vi "Autonomous Independent.vi"   [LabVIEW 2019]
doc: "This VI is called when autonomous begins, and will automatically be terminated when autonomous ends. You can carry out timed or sensor driven robot movement independently without needing to return to the caller."
uses:
  <vilib>/Rock Robotics/WPI/ThirdParty/Phoenix-LabVIEW/Motor Controller/Sensor/CTRE_Phoenix_MotorControl_SetIntegratedSensorPosition_TalonFX.vi
  <vilib>/Rock Robotics/WPI/Solenoid/WPI_SolenoidValue.ctl
  <vilib>/Rock Robotics/WPI/Solenoid/WPI_SolenoidSetEnum.vi
  <vilib>/Rock Robotics/WPI/ThirdParty/Phoenix-LabVIEW/Motor Controller/Controls/CTRE_Phoenix_MotorControl_ControlMode.ctl
  <vilib>/Rock Robotics/Network Tables/NT Write Number.vi
  <vilib>/Rock Robotics/Network Tables/NT Write Numeric Array.vi
  <vilib>/Rock Robotics/Network Tables/NT Read String.vi
panel:
  # "Be sure to right-click and choose Data Operations>>Make Current Value default if you want to save the array values with the VI"
types:
  T1 = typedef "WPI_JoystickDevRef.ctl" = cluster{"Device":T2}
  T2 = typedef "WPI_JoystickDeviceEnum.ctl" = enum16{"USB 0", "USB 1", "USB 2", "USB 3", "USB 4", "USB 5"}
  T3 = typedef "WPI_MotorControlDeviceRef.ctl" = cluster{"DeviceStatus":errorcluster, "Type":T4, "PWM":cluster{"PWM Channel":T5, "DeadBand":T6}, "CAN":cluster{"Device Number":u8, "SetOutput VI Ref":variant, "GetOutput VI Ref":variant, "Enable VI Ref":variant, "Disable VI Ref":variant, "Data":variant}, "Invert":bool, "DIO PWM":cluster{"PWM \"Enable\" Channel":T5, "DIOChannel":T7, "PWM Rate":dbl}}
  T4 = typedef "WPI_MotorControlType.ctl" = enum16{"PWM", "CAN", "DIO PWM"}
  T5 = typedef "FPGA_DIOPWMChannel.ctl" = enum8{"PWM 0", "PWM 1", "PWM 2", "PWM 3", "PWM 4", "PWM 5", "PWM 6", "PWM 7", "PWM 8", "PWM 9", "PWM MXP 0", "PWM MXP 1", "PWM MXP 2", "PWM MXP 3", "PWM MXP 4", "PWM MXP 5", "PWM MXP 6", "PWM MXP 7", "PWM MXP 8", "PWM MXP 9", "Invalid"}
  T6 = typedef "WPI_PWMDeadband.ctl" = cluster{"Name":string, "maxPositivePwm":i32, "minPositivePwm":i32, "centerPwm":i32, "maxNegativePwm":i32, "minNegativePwm":i32, "angularRange":u16}
  T7 = typedef "FPGA_DIOChannel.ctl" = enum8{"DIO 0", "DIO 1", "DIO 2", "DIO 3", "DIO 4", "DIO 5", "DIO 6", "DIO 7", "DIO 8", "DIO 9", "DIO MXP 0", "DIO MXP 1", "DIO MXP 2", "DIO MXP 3", "DIO MXP 4", "DIO MXP 5", "DIO MXP 6", "DIO MXP 7", "DIO MXP 8", "DIO MXP 9", "DIO MXP 10", "DIO MXP 11", "DIO MXP 12", "DIO MXP 13", "DIO MXP 14", "DIO MXP 15", "SPI Port CS1", "SPI Port CS2", "SPI Port CS3", "SPI Port MISO", "SPI Port MOSI", "Invalid"}
  T8 = typedef "WPI_SolenoidDevRef.ctl" = cluster{"DevStatus":errorcluster, "Pneumatics Control Module":u8, "Forward Solenoid Channel":T9, "Reverse Solenoid Channel":T9}
  T9 = typedef "WPI_SolenoidChannel.ctl" = enum8{"Solenoid 0", "Solenoid 1", "Solenoid 2", "Solenoid 3", "Solenoid 4", "Solenoid 5", "Solenoid 6", "Solenoid 7", "Invalid"}
  T10 = typedef "WPI_SolenoidValue.ctl" = enum16{"Off", "On", "Forward", "Reverse"}
  T11 = typedef "CTRE_Phoenix_MotorControl_ControlMode.ctl" = u16
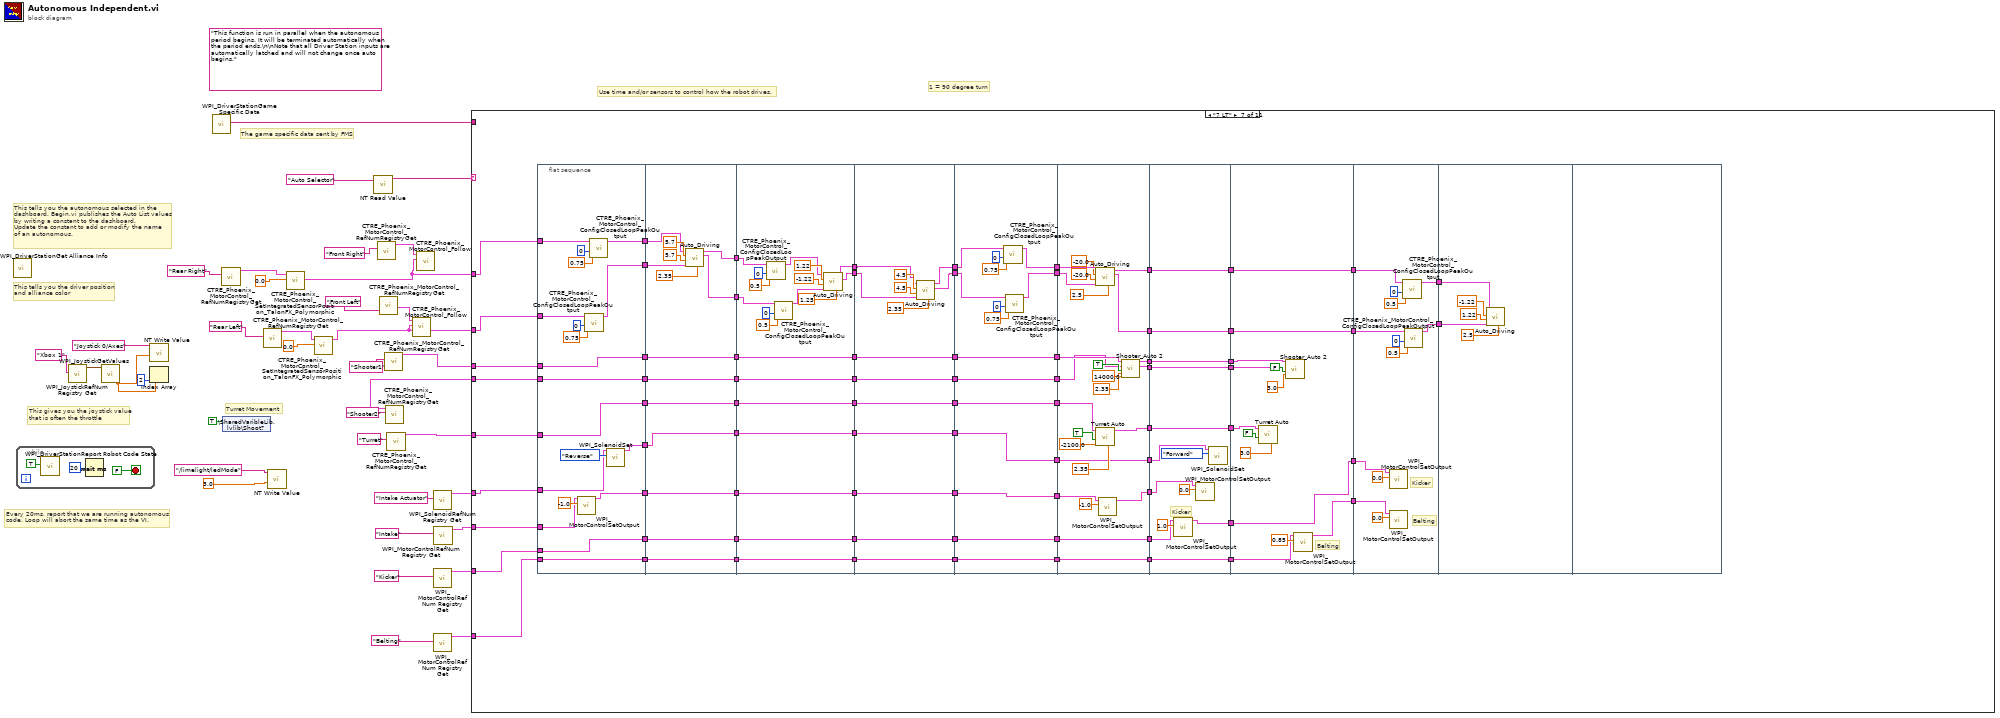
[diagram p0: block diagram]
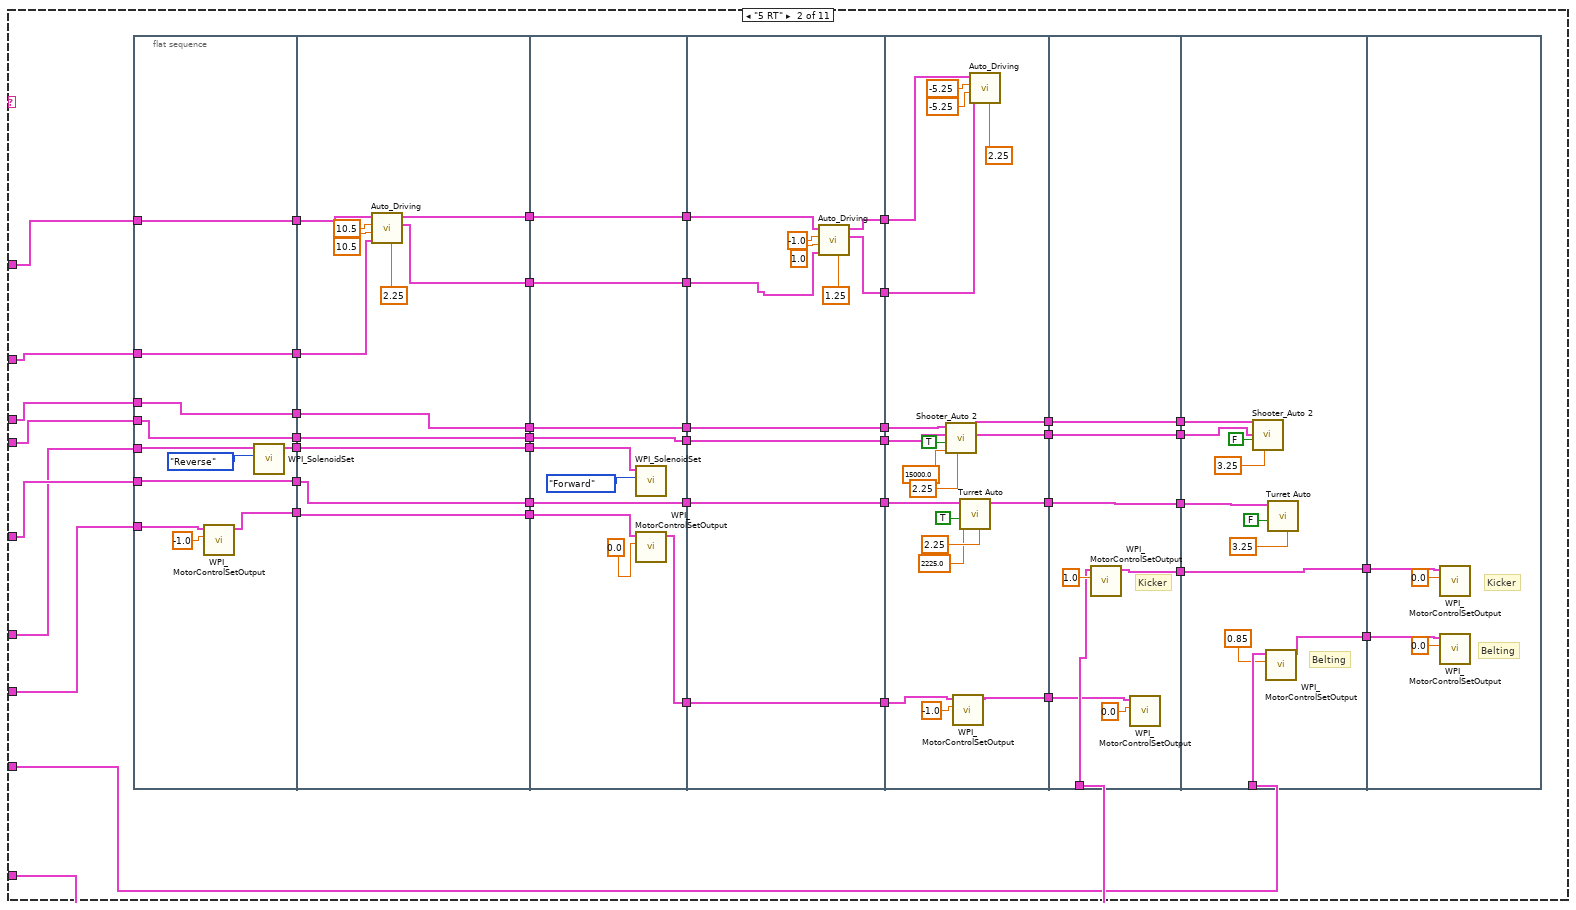
[diagram p3: hidden frame]
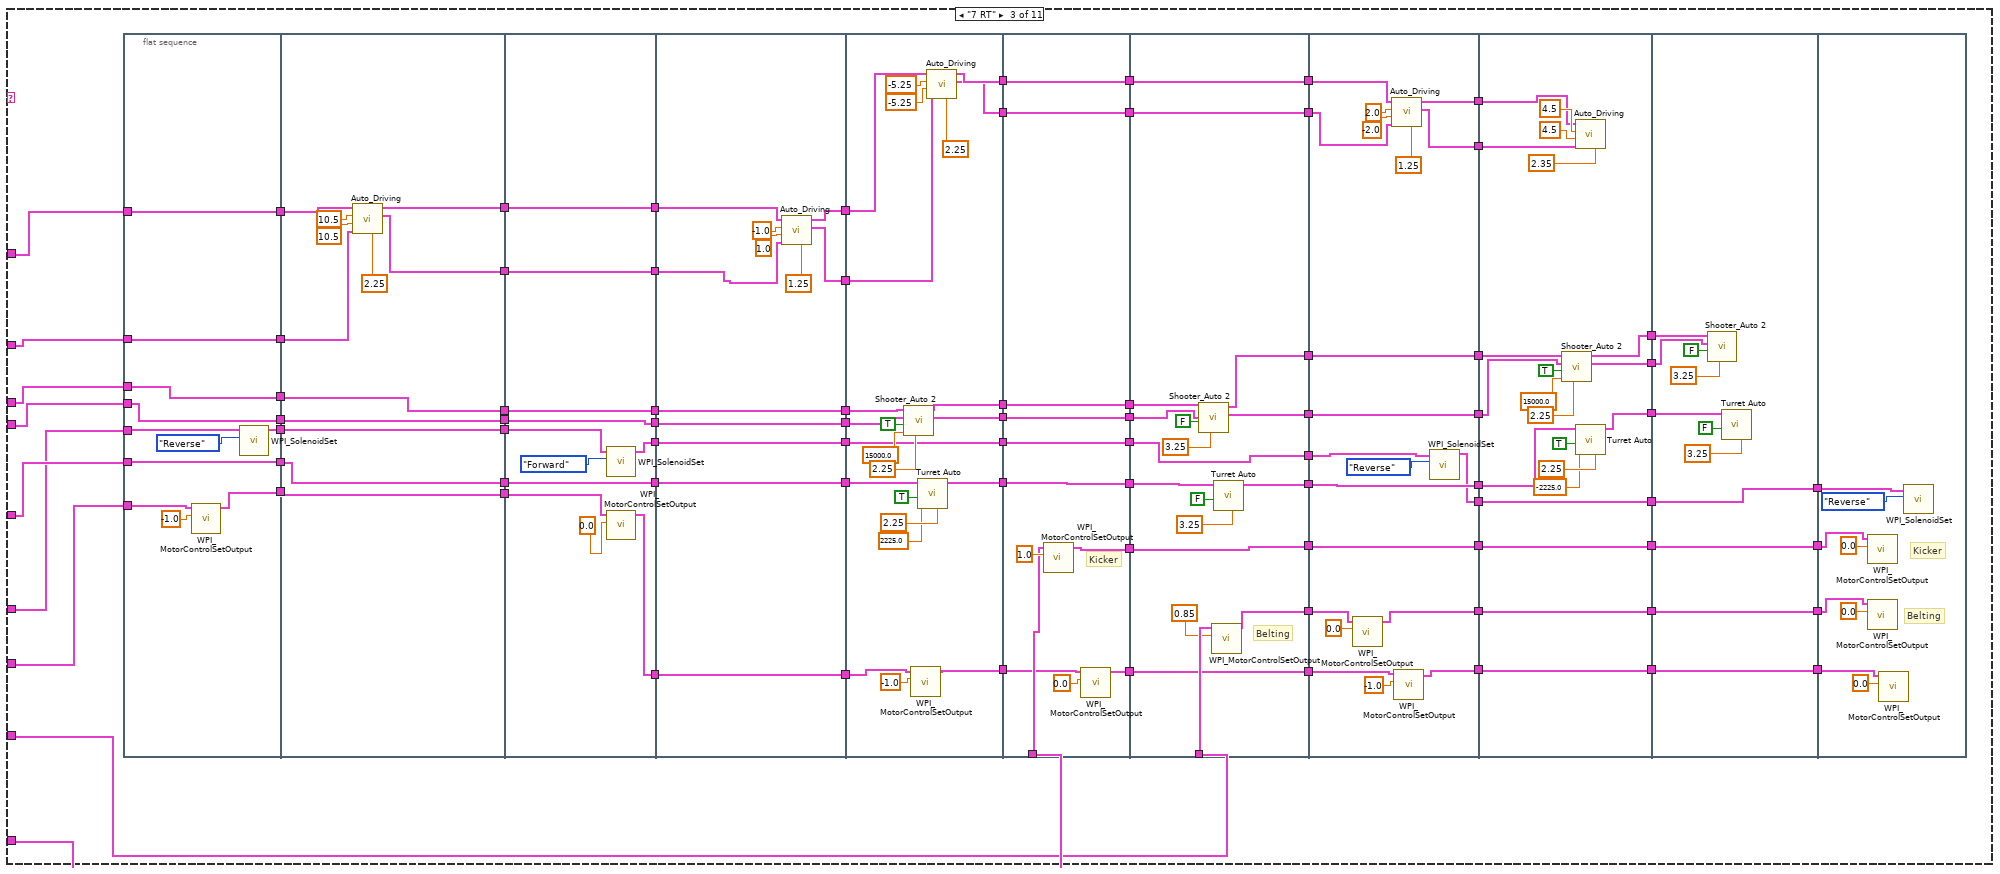
[diagram p4: hidden frame]
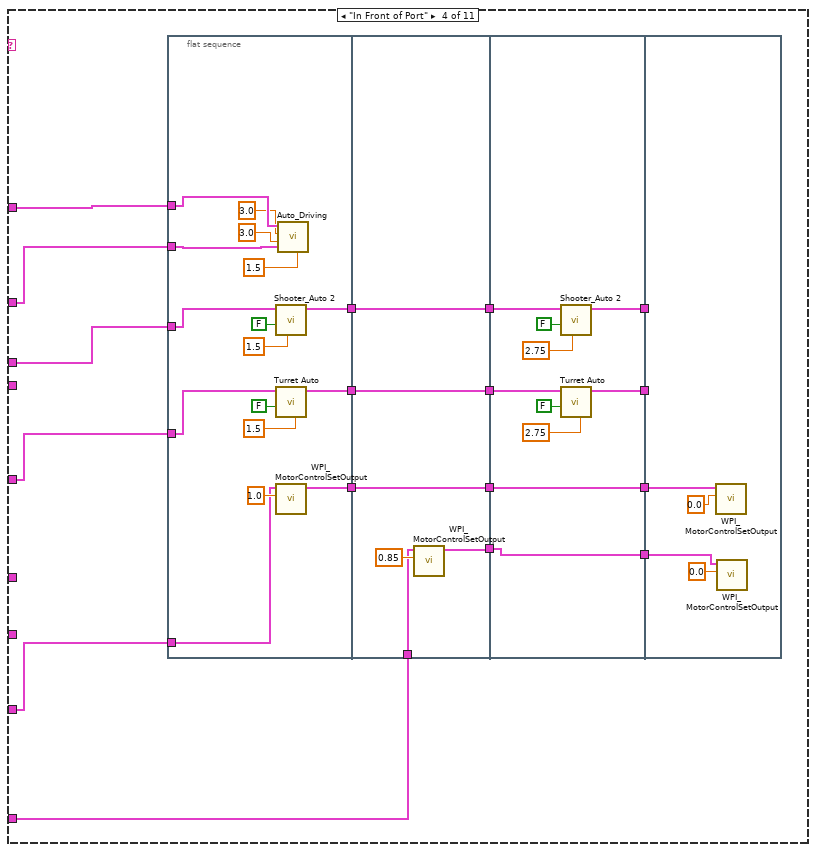
[diagram p5: hidden frame]
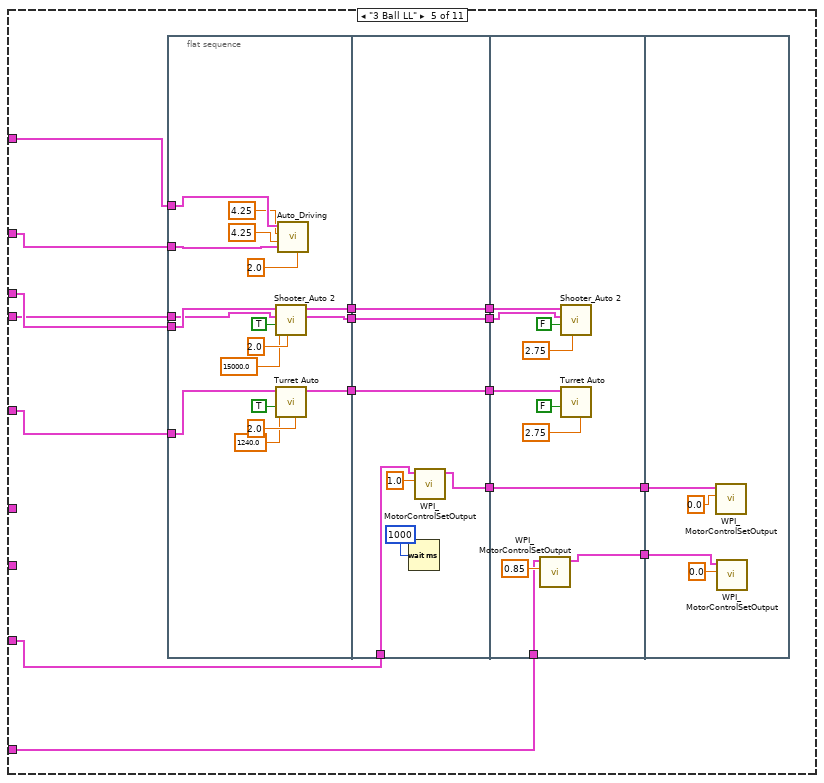
[diagram p6: hidden frame]
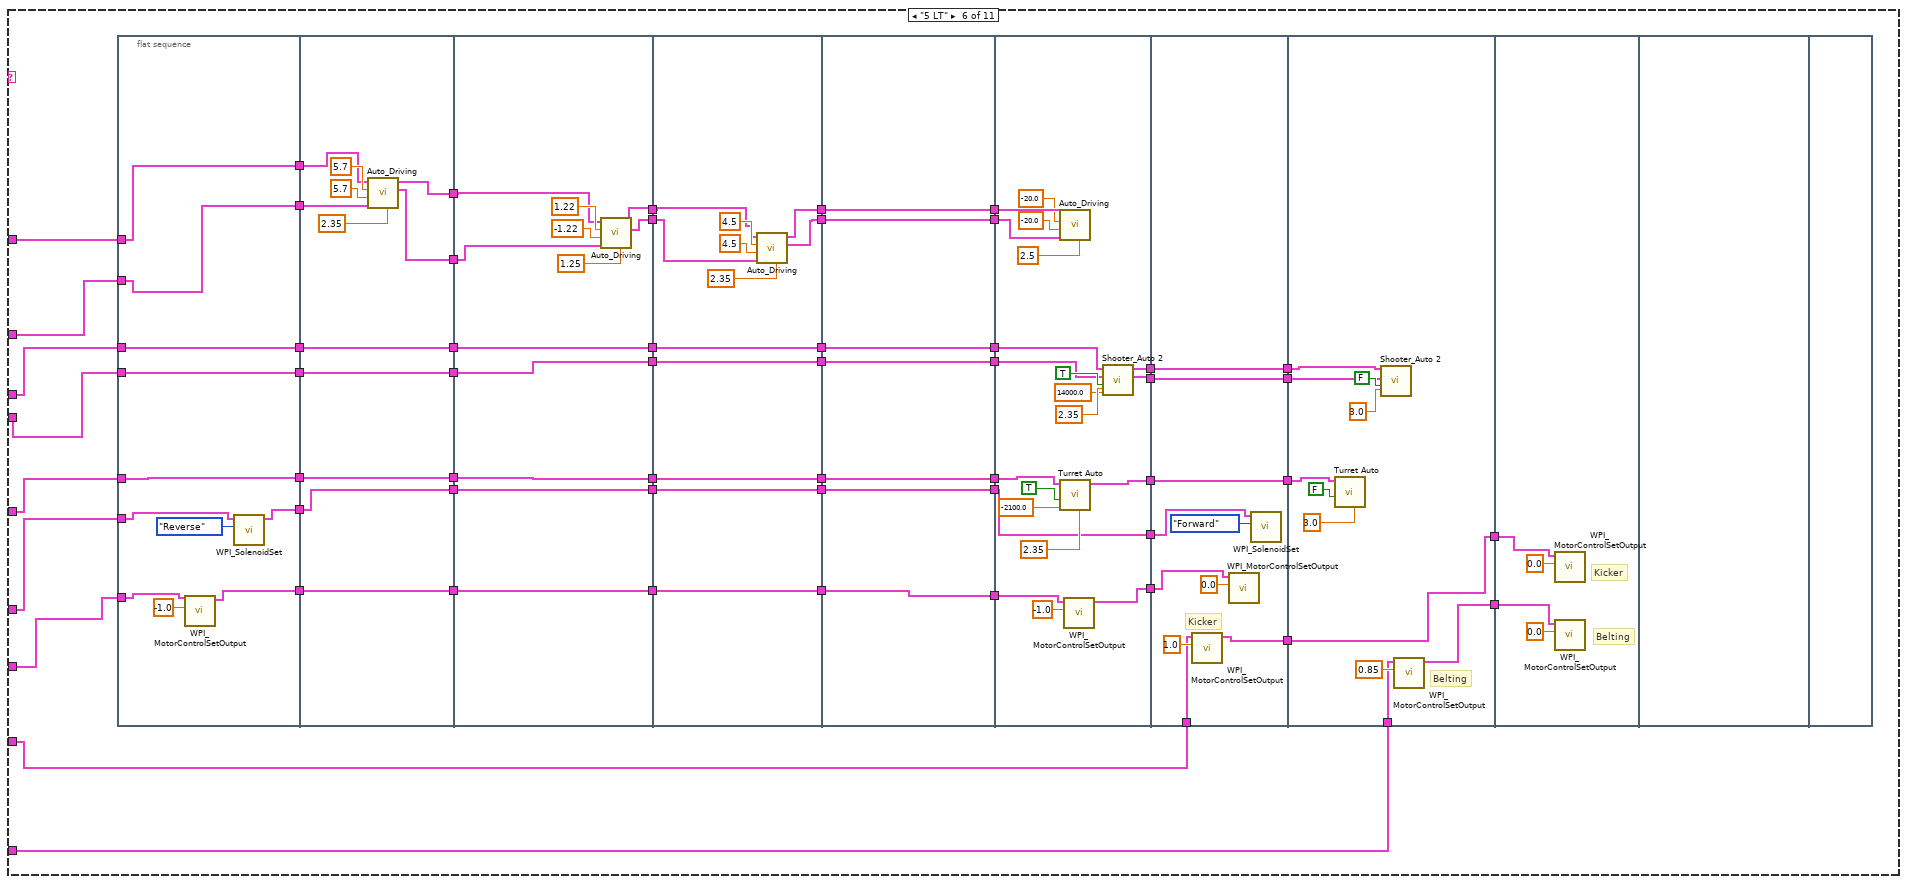
[diagram p7: hidden frame]
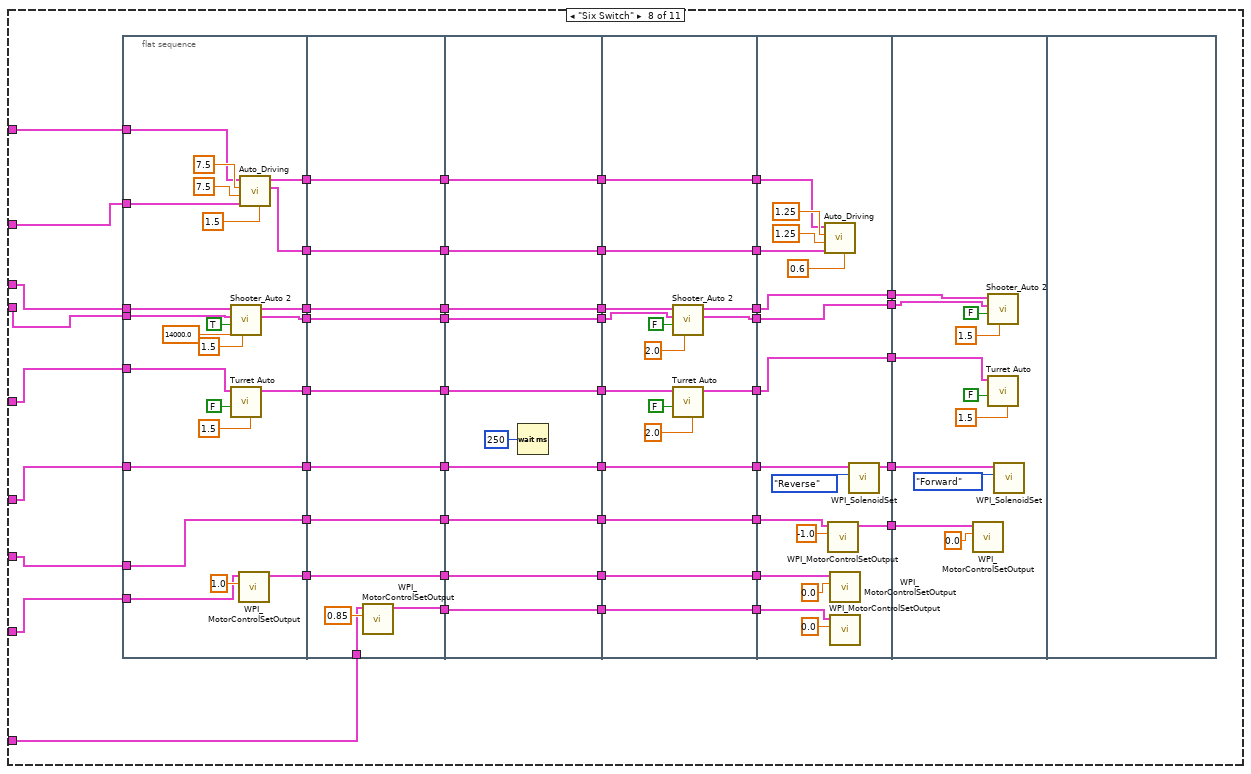
[diagram p8: hidden frame]
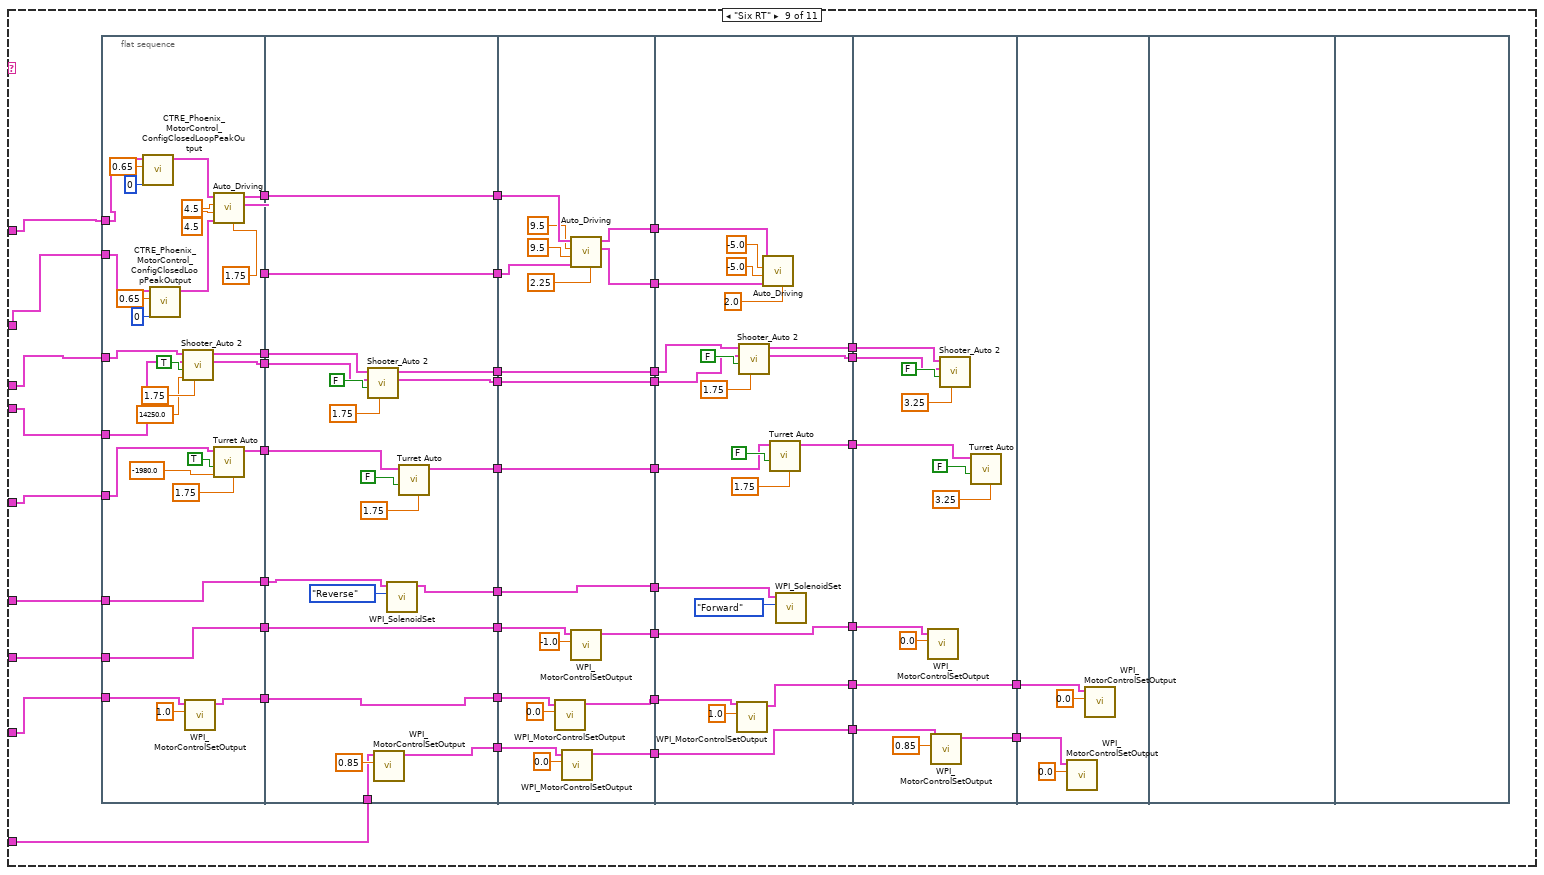
[diagram p9: hidden frame]
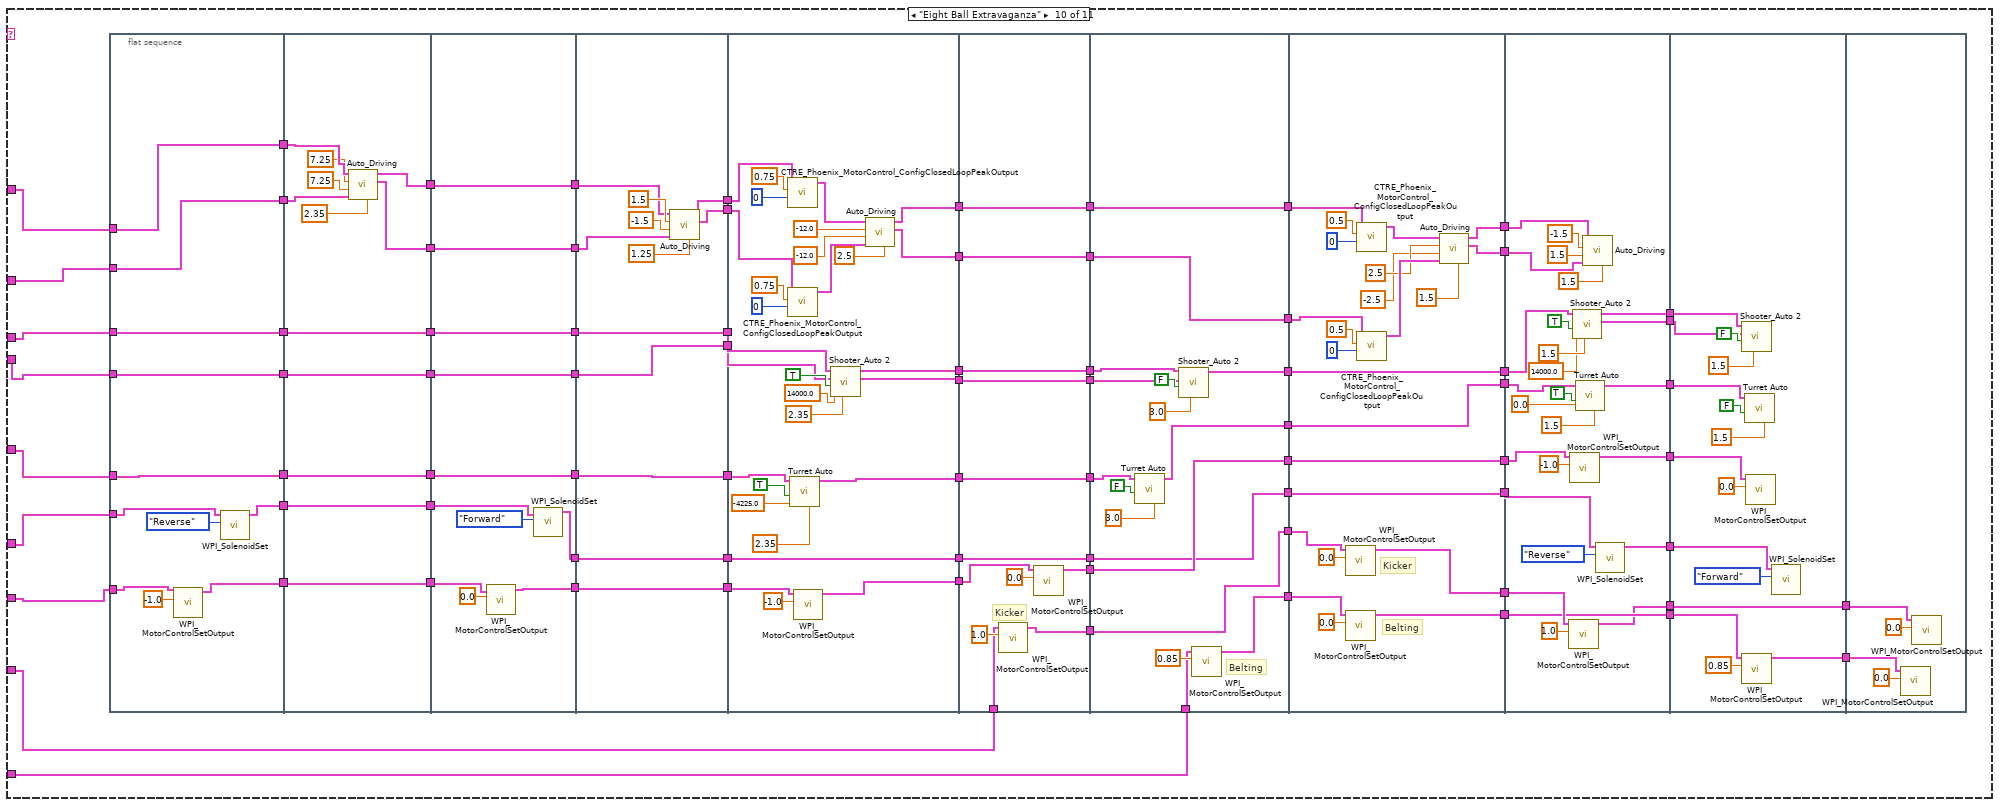
[diagram p10: hidden frame]
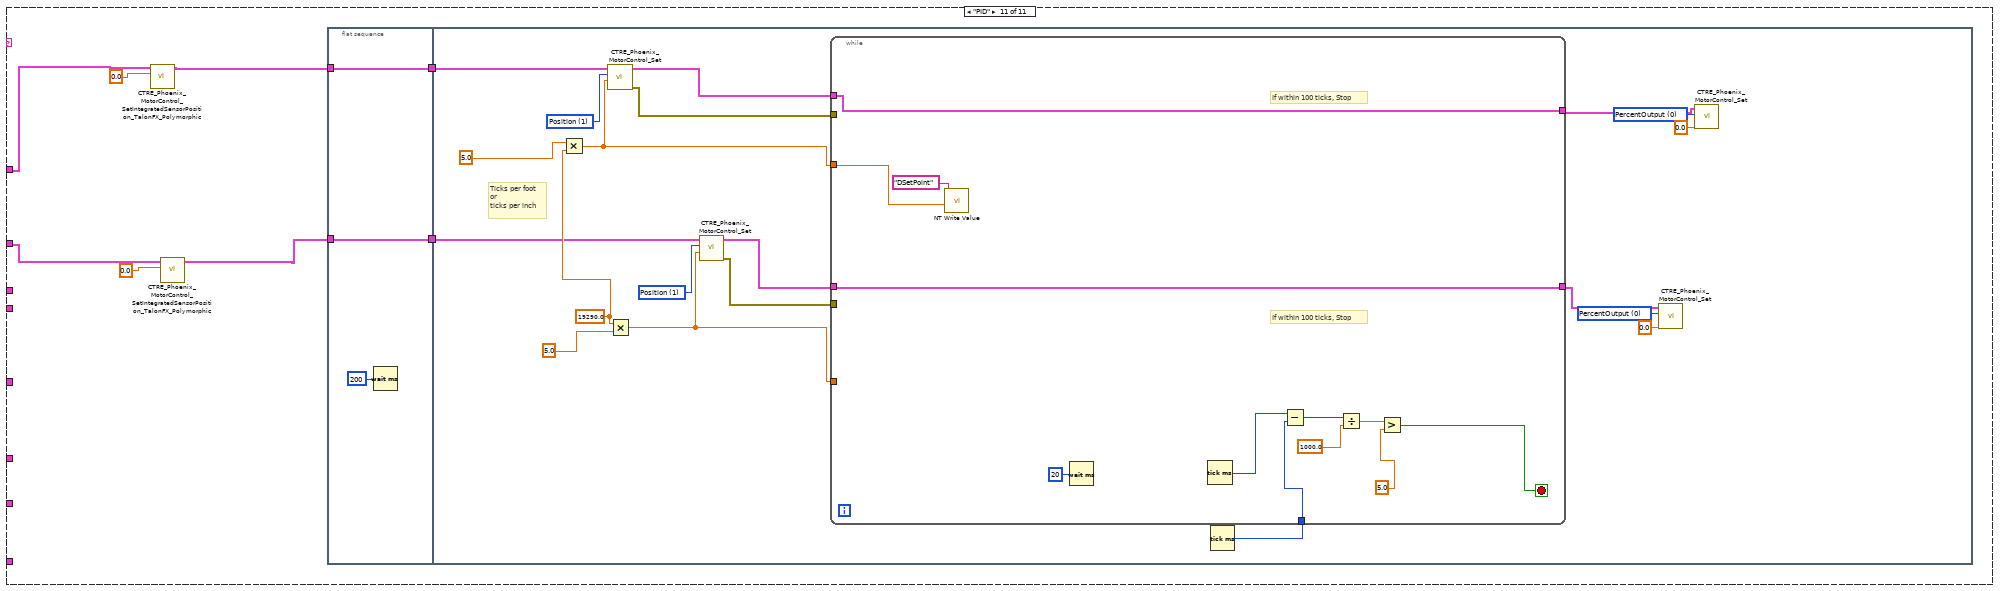
[diagram p11: hidden frame]
diagram:
  (unwired) "This function is run in parallel when the autonomous period begins. It will be terminated automatically when the period ends.\n\nNote that all Driver Station inputs are automatically latched and will not change once auto begins."
  # "1 = 90 degree turn"
  # "Turret Movement"
  # "The game specific data sent by FMS"
  # "This tells you the autonomous selected in the \ndashboard. Begin.vi publishes the Auto List values\nby writing a constant to the dashboard.\nUpdate the constant to add or modify the name\nof an autonomous."
  # "Every 20ms, report that we are running autonomous\ncode. Loop will abort the same time as the VI."
  # "This gives you the joystick value\nthat is often the throttle"
  # "Use time and/or sensors to control how the robot drives."
  # "This tells you the driver position\nand alliance color"
  n1 = call <vilib>:"WPI_DriverStationGet Alliance Info.vi"() -> ()  [unwired: 12 out]
  n2 = while {
    stop <- FALSE stop-if-true
    n3 = call <vilib>:"WPI_DriverStationReport Robot Code State.vi"("Autonomous"=TRUE) -> ()  [unwired: 10 in, 1 out]
    n4 = Wait (ms)(milliseconds to wait=u32 20) -> ()  [unwired: 1 out]
  }
  n5 = call <vilib>:"WPI_JoystickRefNum Registry Get.vi"("refnum name"="Xbox 1") -> ("JoystickDevRef"=w36:T1)  [unwired: 1 in, 9 out]
  n6 = call <vilib>:"WPI_JoystickGetValues.vi"("JoystickDevRef"=w36) -> ("Axes"=w32:dbl[])  [unwired: 6 in, 4 out]
  n7 = call-poly <vilib>:"NT Write Value.vi"("Numeric Array"=w32, "Name"="Joystick 0/Axes") -> ()  [unwired: 9 in, 1 out]
  n8 = Index Array(array=w32, index=2) -> ()  [unwired: 1 out]
  n9 = call <vilib>:"WPI_DriverStationGame Specific Data.vi"() -> ("Game Specific Data"=w30:string)  [unwired: 11 in]
  n10 = call <vilib>:"CTRE_Phoenix_MotorControl_RefNumRegistryGet.vi"("refnum name"="Rear Right") -> ("PhoenixMotorControlDevRef"=w15:T3)  [unwired: 9 in, 1 out]
  n11 = shared-variable ".\\SharedVaribleLib.lvlib\\Shoot?"(TRUE ("Shoot?")) -> ()  [unwired: 1 in, 1 out]
  n12 = call <vilib>:"CTRE_Phoenix_MotorControl_RefNumRegistryGet.vi"("refnum name"="Rear Left") -> ("PhoenixMotorControlDevRef"=w18:T3)  [unwired: 9 in, 1 out]
  n13 = call-poly <vilib>:"NT Write Value.vi"("Numeric"=3.0 ("Default Value"), "Name"="/limelight/ledMode") -> ()  [unwired: 9 in, 1 out]
  n14 = call-poly <vilib>:"CTRE_Phoenix_MotorControl_SetIntegratedSensorPosition_TalonFX_Polymorphic.vi"("New Position"=0.0, "PhoenixMotorControlDevRef"=w15) -> ("PhoenixMotorControlDevRef"=w14:T3)  [unwired: 8 in, 1 out]
  n15 = call-poly <vilib>:"CTRE_Phoenix_MotorControl_SetIntegratedSensorPosition_TalonFX_Polymorphic.vi"("New Position"=0.0, "PhoenixMotorControlDevRef"=w18) -> ("PhoenixMotorControlDevRef"=w17:T3)  [unwired: 8 in, 1 out]
  n16 = call-poly <vilib>:"NT Read Value.vi"("Name"="Auto Selector") -> ("String"=w33:string)  [unwired: 9 in, 1 out]
  n17 = call <vilib>:"CTRE_Phoenix_MotorControl_RefNumRegistryGet.vi"("refnum name"="Front Right") -> ("PhoenixMotorControlDevRef"=w3:T3)  [unwired: 9 in, 1 out]
  n18 = call <vilib>:"CTRE_Phoenix_MotorControl_RefNumRegistryGet.vi"("refnum name"="Front Left") -> ("PhoenixMotorControlDevRef"=w25:T3)  [unwired: 9 in, 1 out]
  n19 = call <vilib>:"CTRE_Phoenix_MotorControl_RefNumRegistryGet.vi"("refnum name"="Shooter1") -> ("PhoenixMotorControlDevRef"=w5:T3)  [unwired: 9 in, 1 out]
  n20 = call <vilib>:"CTRE_Phoenix_MotorControl_RefNumRegistryGet.vi"("refnum name"="Shooter2") -> ("PhoenixMotorControlDevRef"=w4:T3)  [unwired: 9 in, 1 out]
  n21 = call <vilib>:"CTRE_Phoenix_MotorControl_RefNumRegistryGet.vi"("refnum name"="Turret") -> ("PhoenixMotorControlDevRef"=w20:T3)  [unwired: 9 in, 1 out]
  n22 = call <vilib>:"CTRE_Phoenix_MotorControl_Follow.vi"("Master Controller to Follow"=w17, "PhoenixMotorControlDevRef"=w25) -> ()  [unwired: 8 in, 2 out]
  n23 = call <vilib>:"CTRE_Phoenix_MotorControl_Follow.vi"("Master Controller to Follow"=w14, "PhoenixMotorControlDevRef"=w3) -> ()  [unwired: 8 in, 2 out]
  n24 = call <vilib>:"WPI_SolenoidRefNum Registry Get.vi"("refnum name"="Intake Actuator") -> ("SolenoidDevRef"=w11:T8)  [unwired: 9 in, 1 out]
  n25 = call <vilib>:"WPI_MotorControlRefNum Registry Get.vi"("refnum name"="Kicker") -> ("MotorControlDevRef"=w7:T3)  [unwired: 9 in, 1 out]
  n26 = call <vilib>:"WPI_MotorControlRefNum Registry Get.vi"("refnum name"="Belting") -> ("MotorControlDevRef"=w6:T3)  [unwired: 9 in, 1 out]
  n27 = call <vilib>:"WPI_MotorControlRefNum Registry Get.vi"("refnum name"="Intake") -> ("MotorControlDevRef"=w10:T3)  [unwired: 9 in, 1 out]
  n28 = case shown="\"7 LT\"" w33 {
    tunnel: w30 -> [_ _ _ _ _ _ _ _ _ _ _]
    tunnel: w17 -> [_ w76 w244 w428 w473 w573 w720 w941 w1081 w1226 w1443]
    tunnel: w14 -> [_ w85 w253 w429 w474 w574 w719 w940 w1082 w1227 w1444]
    tunnel: w20 -> [_ w84 w252 w427 w471 w569 w684 w939 w1078 w1230 _]
    tunnel: w11 -> [_ w83 w251 _ _ w575 w718 w926 w1061 w1229 _]
    tunnel: w10 -> [_ w61 w231 _ _ w523 w717 w929 w1063 w1228 _]
    tunnel: w7 -> [_ w41 w211 w414 w466 w553 w710 w937 w1077 w1225 _]
    tunnel: w6 -> [_ w42 w212 w421 w467 w568 w702 w936 w1072 w1224 _]
    tunnel: w5 -> [_ w60 w230 w426 w472 w565 w696 w942 w1079 w1232 _]
    tunnel: w4 -> [_ w52 w222 _ w470 w562 w690 w943 w1080 w1231 _]
    frame Default {
    }
    frame "5 RT" {
      n29 = flat-sequence {
        tunnel: w76 -> [w94]
        tunnel: w83 -> [w90]
        tunnel: w84 -> [w95]
        tunnel: w85 -> [w96]
        tunnel: [w96] -> w73
        tunnel: [w95] -> w72
        tunnel: [w94] -> w71
        tunnel: [w92] -> w70
        tunnel: [w89] -> w68
        tunnel: w61 -> [w88]
        tunnel: w60 -> [w87]
        tunnel: [w87] -> w59
        tunnel: w52 -> [w86]
        tunnel: [w86] -> w48
        tunnel: [w104] -> w81
        tunnel: [w103] -> w79
        tunnel: [w100] -> w77
        tunnel: w73 -> [w108]
        tunnel: w72 -> [w100]
        tunnel: w71 -> [w102]
        tunnel: w70 -> [w99]
        tunnel: [w101] -> w69
        tunnel: w68 -> [w101]
        tunnel: [w99] -> w67
        tunnel: w59 -> [w98]
        tunnel: [w98] -> w58
        tunnel: [w97] -> w49
        tunnel: w48 -> [w97]
        tunnel: [w116] -> w82
        tunnel: w81 -> [w116]
        tunnel: [w115] -> w80
        tunnel: w79 -> [w115]
        tunnel: [w114] -> w78
        tunnel: w77 -> [w114]
        tunnel: w69 -> [w112]
        tunnel: w67 -> [w113]
        tunnel: w58 -> [w111]
        tunnel: [w111] -> w57
        tunnel: [w110] -> w50
        tunnel: w49 -> [w110]
        tunnel: [w109] -> w44
        tunnel: w82 -> [w119]
        tunnel: w80 -> [w120]
        tunnel: [w126] -> w56
        tunnel: [w125] -> w55
        tunnel: [w124] -> w54
        tunnel: w78 -> [w124]
        tunnel: w57 -> [w123]
        tunnel: [w123] -> w53
        tunnel: [w122] -> w51
        tunnel: w50 -> [w122]
        tunnel: [w121] -> w45
        tunnel: w44 -> [w121]
        tunnel: w56 -> [w142]
        tunnel: w55 -> [w146]
        tunnel: w54 -> [w145]
        tunnel: [w143] -> w66
        tunnel: [w139] -> w64
        tunnel: w53 -> [w138]
        tunnel: w51 -> [w134]
        tunnel: [w133] -> w46
        tunnel: w45 -> [w132]
        tunnel: [w130] -> w43
        tunnel: w66 -> [w157]
        tunnel: [w157] -> w65
        tunnel: w64 -> [w156]
        tunnel: [w156] -> w63
        tunnel: [w154] -> w62
        tunnel: w42 -> [w153]
        tunnel: [w152] -> w47
        tunnel: w46 -> [w152]
        tunnel: w43 -> [w150]
        tunnel: w65 -> [w168]
        tunnel: w63 -> [w165]
        tunnel: [w162] -> w75
        tunnel: [w164] -> w74
        tunnel: w62 -> [w164]
        tunnel: w41 -> [w163]
        tunnel: w47 -> [w158]
        tunnel: w75 -> [w170]
        tunnel: w74 -> [w169]
        frame #0 {
          n30 = call <vilib>:"WPI_MotorControlSetOutput.vi"("Output"=-1.0, "MotorControlDevRef"=w88) -> ("MotorControlDevRef"=w92:T3)  [unwired: 7 in, 2 out]
          n31 = call-poly <vilib>:"WPI_SolenoidSet.vi"("Value"=WPI_SolenoidValue."Reverse", "SolenoidDevRef"=w90) -> ("SolenoidDevRef"=w89:T8)  [unwired: 8 in, 1 out]
        }
        frame #1 {
          n32 = call "Auto_Driving.vi"("MaxTime"=2.25, "Motor2Ref"=w102, "Motor2Distance"=10.5, "Motor1Distance"=10.5, "Motor1Ref"=w108) -> ("Motor Bottom Out"=w103:T3, "Motor Top Out"=w104:T3)  [unwired: 4 in, 1 out]
        }
        frame #2 {
          n33 = call-poly <vilib>:"WPI_SolenoidSet.vi"("Value"=WPI_SolenoidValue."Forward", "SolenoidDevRef"=w112) -> ()  [unwired: 8 in, 2 out]
          n34 = call <vilib>:"WPI_MotorControlSetOutput.vi"("Output"=0.0, "MotorControlDevRef"=w113) -> ("MotorControlDevRef"=w109:T3)  [unwired: 7 in, 2 out]
        }
        frame #3 {
          n35 = call "Auto_Driving.vi"("MaxTime"=1.25, "Motor2Ref"=w120, "Motor2Distance"=1.0, "Motor1Distance"=-1.0, "Motor1Ref"=w119) -> ("Motor Bottom Out"=w126:T3, "Motor Top Out"=w125:T3)  [unwired: 4 in, 1 out]
        }
        frame #4 {
          n36 = call "Shooter_Auto 2.vi"("RunTime"=2.25, "RPM Override"=15000.0, "Override?"=TRUE, "Followers"=w134, "Master"=w138) -> ("Follower"=w133:T3, "Master"=w139:T3)  [unwired: 5 in]
          n37 = call <vilib>:"WPI_MotorControlSetOutput.vi"("Output"=-1.0, "MotorControlDevRef"=w132) -> ("MotorControlDevRef"=w130:T3)  [unwired: 7 in, 2 out]
          n38 = call "Turret Auto.vi"("RunTime"=2.25, "Override_Value"=2225.0, "Overide"=TRUE, "Motor1Ref"=w145) -> ("PhoenixMotorControlDevRef"=w143:T3)  [unwired: 7 in]
          n39 = call "Auto_Driving.vi"("MaxTime"=2.25, "Motor2Ref"=w142, "Motor2Distance"=-5.25, "Motor1Distance"=-5.25, "Motor1Ref"=w146) -> ()  [unwired: 4 in, 3 out]
        }
        frame #5 {
          # "Kicker"
          n40 = call <vilib>:"WPI_MotorControlSetOutput.vi"("Output"=1.0, "MotorControlDevRef"=w153) -> ("MotorControlDevRef"=w154:T3)  [unwired: 7 in, 2 out]
          n41 = call <vilib>:"WPI_MotorControlSetOutput.vi"("Output"=0.0, "MotorControlDevRef"=w150) -> ()  [unwired: 7 in, 3 out]
        }
        frame #6 {
          # "Belting"
          n42 = call "Shooter_Auto 2.vi"("RunTime"=3.25, "Override?"=FALSE, "Followers"=w158, "Master"=w165) -> ()  [unwired: 6 in, 2 out]
          n43 = call <vilib>:"WPI_MotorControlSetOutput.vi"("Output"=0.85, "MotorControlDevRef"=w163) -> ("MotorControlDevRef"=w162:T3)  [unwired: 7 in, 2 out]
          n44 = call "Turret Auto.vi"("RunTime"=3.25, "Overide"=FALSE, "Motor1Ref"=w168) -> ()  [unwired: 8 in, 1 out]
        }
        frame #7 {
          # "Belting"
          # "Kicker"
          n45 = call <vilib>:"WPI_MotorControlSetOutput.vi"("Output"=0.0, "MotorControlDevRef"=w169) -> ()  [unwired: 7 in, 3 out]
          n46 = call <vilib>:"WPI_MotorControlSetOutput.vi"("Output"=0.0, "MotorControlDevRef"=w170) -> ()  [unwired: 7 in, 3 out]
        }
      }
    }
    frame "7 RT" {
      n47 = flat-sequence {
        tunnel: w244 -> [w262]
        tunnel: w251 -> [w258]
        tunnel: w252 -> [w263]
        tunnel: w253 -> [w264]
        tunnel: [w264] -> w243
        tunnel: [w263] -> w242
        tunnel: [w262] -> w241
        tunnel: [w260] -> w240
        tunnel: [w257] -> w238
        tunnel: w231 -> [w256]
        tunnel: w230 -> [w255]
        tunnel: [w255] -> w229
        tunnel: w222 -> [w254]
        tunnel: [w254] -> w218
        tunnel: [w272] -> w249
        tunnel: [w271] -> w247
        tunnel: [w268] -> w245
        tunnel: w243 -> [w276]
        tunnel: w242 -> [w268]
        tunnel: w241 -> [w270]
        tunnel: w240 -> [w267]
        tunnel: [w269] -> w239
        tunnel: w238 -> [w269]
        tunnel: [w267] -> w237
        tunnel: w229 -> [w266]
        tunnel: [w266] -> w228
        tunnel: [w265] -> w219
        tunnel: w218 -> [w265]
        tunnel: [w285] -> w250
        tunnel: w249 -> [w285]
        tunnel: [w284] -> w248
        tunnel: w247 -> [w284]
        tunnel: [w283] -> w246
        tunnel: w245 -> [w283]
        tunnel: w239 -> [w281]
        tunnel: w237 -> [w282]
        tunnel: w228 -> [w280]
        tunnel: [w280] -> w227
        tunnel: [w279] -> w220
        tunnel: w219 -> [w279]
        tunnel: [w278] -> w214
        tunnel: [w277] -> w192
        tunnel: w250 -> [w289]
        tunnel: w248 -> [w290]
        tunnel: [w296] -> w226
        tunnel: [w295] -> w225
        tunnel: [w294] -> w224
        tunnel: w246 -> [w294]
        tunnel: w227 -> [w293]
        tunnel: [w293] -> w223
        tunnel: [w292] -> w221
        tunnel: w220 -> [w292]
        tunnel: [w291] -> w215
        tunnel: w214 -> [w291]
        tunnel: [w288] -> w193
        tunnel: w192 -> [w288]
        tunnel: w226 -> [w315]
        tunnel: w225 -> [w319]
        tunnel: w224 -> [w318]
        tunnel: [w316] -> w236
        tunnel: [w312] -> w234
        tunnel: w223 -> [w311]
        tunnel: w221 -> [w307]
        tunnel: [w306] -> w216
        tunnel: w215 -> [w305]
        tunnel: [w303] -> w213
        tunnel: [w302] -> w202
        tunnel: [w301] -> w199
        tunnel: [w300] -> w194
        tunnel: w193 -> [w300]
        tunnel: w236 -> [w334]
        tunnel: [w334] -> w235
        tunnel: w234 -> [w333]
        tunnel: [w333] -> w233
        tunnel: [w331] -> w232
        tunnel: w212 -> [w330]
        tunnel: [w329] -> w217
        tunnel: w216 -> [w329]
        tunnel: w213 -> [w327]
        tunnel: [w326] -> w203
        tunnel: w202 -> [w326]
        tunnel: [w325] -> w200
        tunnel: w199 -> [w325]
        tunnel: [w324] -> w195
        tunnel: w194 -> [w324]
        tunnel: [w323] -> w190
        tunnel: w235 -> [w352]
        tunnel: w233 -> [w349]
        tunnel: [w346] -> w210
        tunnel: [w348] -> w209
        tunnel: w232 -> [w348]
        tunnel: w211 -> [w347]
        tunnel: w217 -> [w342]
        tunnel: [w341] -> w204
        tunnel: w203 -> [w341]
        tunnel: [w340] -> w201
        tunnel: w200 -> [w340]
        tunnel: [w339] -> w196
        tunnel: w195 -> [w339]
        tunnel: [w338] -> w191
        tunnel: w190 -> [w338]
        tunnel: [w337] -> w189
        tunnel: [w336] -> w186
        tunnel: [w335] -> w185
        tunnel: w210 -> [w367]
        tunnel: [w366] -> w208
        tunnel: w209 -> [w372]
        tunnel: [w372] -> w206
        tunnel: w204 -> [w365]
        tunnel: w201 -> [w364]
        tunnel: [w363] -> w198
        tunnel: [w362] -> w197
        tunnel: w196 -> [w360]
        tunnel: w191 -> [w358]
        tunnel: w189 -> [w357]
        tunnel: [w357] -> w188
        tunnel: [w356] -> w187
        tunnel: w186 -> [w356]
        tunnel: w185 -> [w355]
        tunnel: [w355] -> w184
        tunnel: [w354] -> w178
        tunnel: [w353] -> w173
        tunnel: w208 -> [w393]
        tunnel: [w393] -> w207
        tunnel: w206 -> [w392]
        tunnel: [w392] -> w205
        tunnel: w198 -> [w388]
        tunnel: w197 -> [w387]
        tunnel: w188 -> [w380]
        tunnel: w187 -> [w379]
        tunnel: w184 -> [w378]
        tunnel: [w377] -> w183
        tunnel: [w376] -> w182
        tunnel: [w375] -> w181
        tunnel: w178 -> [w374]
        tunnel: [w374] -> w177
        tunnel: [w373] -> w174
        tunnel: w173 -> [w373]
        tunnel: w207 -> [w397]
        tunnel: w205 -> [w396]
        tunnel: w183 -> [w400]
        tunnel: w182 -> [w399]
        tunnel: w181 -> [w398]
        tunnel: [w397] -> w180
        tunnel: [w396] -> w179
        tunnel: w177 -> [w395]
        tunnel: [w395] -> w176
        tunnel: [w394] -> w175
        tunnel: w174 -> [w394]
        tunnel: w180 -> [w411]
        tunnel: w179 -> [w409]
        tunnel: w176 -> [w407]
        tunnel: w175 -> [w405]
        frame #0 {
          n48 = call <vilib>:"WPI_MotorControlSetOutput.vi"("Output"=-1.0, "MotorControlDevRef"=w256) -> ("MotorControlDevRef"=w260:T3)  [unwired: 7 in, 2 out]
          n49 = call-poly <vilib>:"WPI_SolenoidSet.vi"("Value"=WPI_SolenoidValue."Reverse", "SolenoidDevRef"=w258) -> ("SolenoidDevRef"=w257:T8)  [unwired: 8 in, 1 out]
        }
        frame #1 {
          n50 = call "Auto_Driving.vi"("MaxTime"=2.25, "Motor2Ref"=w270, "Motor2Distance"=10.5, "Motor1Distance"=10.5, "Motor1Ref"=w276) -> ("Motor Bottom Out"=w271:T3, "Motor Top Out"=w272:T3)  [unwired: 4 in, 1 out]
        }
        frame #2 {
          n51 = call-poly <vilib>:"WPI_SolenoidSet.vi"("Value"=WPI_SolenoidValue."Forward", "SolenoidDevRef"=w281) -> ("SolenoidDevRef"=w277:T8)  [unwired: 8 in, 1 out]
          n52 = call <vilib>:"WPI_MotorControlSetOutput.vi"("Output"=0.0, "MotorControlDevRef"=w282) -> ("MotorControlDevRef"=w278:T3)  [unwired: 7 in, 2 out]
        }
        frame #3 {
          n53 = call "Auto_Driving.vi"("MaxTime"=1.25, "Motor2Ref"=w290, "Motor2Distance"=1.0, "Motor1Distance"=-1.0, "Motor1Ref"=w289) -> ("Motor Bottom Out"=w296:T3, "Motor Top Out"=w295:T3)  [unwired: 4 in, 1 out]
        }
        frame #4 {
          n54 = call "Shooter_Auto 2.vi"("RunTime"=2.25, "RPM Override"=15000.0, "Override?"=TRUE, "Followers"=w307, "Master"=w311) -> ("Follower"=w306:T3, "Master"=w312:T3)  [unwired: 5 in]
          n55 = call <vilib>:"WPI_MotorControlSetOutput.vi"("Output"=-1.0, "MotorControlDevRef"=w305) -> ("MotorControlDevRef"=w303:T3)  [unwired: 7 in, 2 out]
          n56 = call "Turret Auto.vi"("RunTime"=2.25, "Override_Value"=2225.0, "Overide"=TRUE, "Motor1Ref"=w318) -> ("PhoenixMotorControlDevRef"=w316:T3)  [unwired: 7 in]
          n57 = call "Auto_Driving.vi"("MaxTime"=2.25, "Motor2Ref"=w315, "Motor2Distance"=-5.25, "Motor1Distance"=-5.25, "Motor1Ref"=w319) -> ("Motor Bottom Out"=w301:T3, "Motor Top Out"=w302:T3)  [unwired: 4 in, 1 out]
        }
        frame #5 {
          # "Kicker"
          n58 = call <vilib>:"WPI_MotorControlSetOutput.vi"("Output"=1.0, "MotorControlDevRef"=w330) -> ("MotorControlDevRef"=w331:T3)  [unwired: 7 in, 2 out]
          n59 = call <vilib>:"WPI_MotorControlSetOutput.vi"("Output"=0.0, "MotorControlDevRef"=w327) -> ("MotorControlDevRef"=w323:T3)  [unwired: 7 in, 2 out]
        }
        frame #6 {
          # "Belting"
          n60 = call "Shooter_Auto 2.vi"("RunTime"=3.25, "Override?"=FALSE, "Followers"=w342, "Master"=w349) -> ("Follower"=w335:T3, "Master"=w336:T3)  [unwired: 6 in]
          n61 = call <vilib>:"WPI_MotorControlSetOutput.vi"("Output"=0.85, "MotorControlDevRef"=w347) -> ("MotorControlDevRef"=w346:T3)  [unwired: 7 in, 2 out]
          n62 = call "Turret Auto.vi"("RunTime"=3.25, "Overide"=FALSE, "Motor1Ref"=w352) -> ("PhoenixMotorControlDevRef"=w337:T3)  [unwired: 8 in]
        }
        frame #7 {
          n63 = call <vilib>:"WPI_MotorControlSetOutput.vi"("Output"=0.0, "MotorControlDevRef"=w367) -> ("MotorControlDevRef"=w366:T3)  [unwired: 7 in, 2 out]
          n64 = call "Auto_Driving.vi"("MaxTime"=1.25, "Motor2Ref"=w364, "Motor2Distance"=-2.0, "Motor1Distance"=2.0, "Motor1Ref"=w365) -> ("Motor Bottom Out"=w362:T3, "Motor Top Out"=w363:T3)  [unwired: 4 in, 1 out]
          n65 = call <vilib>:"WPI_MotorControlSetOutput.vi"("Output"=-1.0, "MotorControlDevRef"=w358) -> ("MotorControlDevRef"=w354:T3)  [unwired: 7 in, 2 out]
          n66 = call-poly <vilib>:"WPI_SolenoidSet.vi"("Value"=WPI_SolenoidValue."Reverse", "SolenoidDevRef"=w360) -> ("SolenoidDevRef"=w353:T8)  [unwired: 8 in, 1 out]
        }
        frame #8 {
          n67 = call "Shooter_Auto 2.vi"("RunTime"=2.25, "RPM Override"=15000.0, "Override?"=TRUE, "Followers"=w378, "Master"=w379) -> ("Follower"=w376:T3, "Master"=w377:T3)  [unwired: 5 in]
          n68 = call "Auto_Driving.vi"("MaxTime"=2.35, "Motor2Ref"=w387, "Motor2Distance"=4.5, "Motor1Distance"=4.5, "Motor1Ref"=w388) -> ()  [unwired: 4 in, 3 out]
          n69 = call "Turret Auto.vi"("RunTime"=2.25, "Override_Value"=-2225.0, "Overide"=TRUE, "Motor1Ref"=w380) -> ("PhoenixMotorControlDevRef"=w375:T3)  [unwired: 7 in]
        }
        frame #9 {
          n70 = call "Shooter_Auto 2.vi"("RunTime"=3.25, "Override?"=FALSE, "Followers"=w399, "Master"=w400) -> ()  [unwired: 6 in, 2 out]
          n71 = call "Turret Auto.vi"("RunTime"=3.25, "Overide"=FALSE, "Motor1Ref"=w398) -> ()  [unwired: 8 in, 1 out]
        }
        frame #10 {
          # "Belting"
          # "Kicker"
          n72 = call <vilib>:"WPI_MotorControlSetOutput.vi"("Output"=0.0, "MotorControlDevRef"=w409) -> ()  [unwired: 7 in, 3 out]
          n73 = call <vilib>:"WPI_MotorControlSetOutput.vi"("Output"=0.0, "MotorControlDevRef"=w411) -> ()  [unwired: 7 in, 3 out]
          n74 = call <vilib>:"WPI_MotorControlSetOutput.vi"("Output"=0.0, "MotorControlDevRef"=w407) -> ()  [unwired: 7 in, 3 out]
          n75 = call-poly <vilib>:"WPI_SolenoidSet.vi"("Value"=WPI_SolenoidValue."Reverse", "SolenoidDevRef"=w405) -> ()  [unwired: 8 in, 2 out]
        }
      }
    }
    frame "In Front of Port" {
      n76 = flat-sequence {
        tunnel: w429 -> [w445]
        tunnel: w428 -> [w444]
        tunnel: w427 -> [w438]
        tunnel: w426 -> [w437]
        tunnel: [w436] -> w425
        tunnel: [w435] -> w423
        tunnel: w414 -> [w431]
        tunnel: [w430] -> w413
        tunnel: w425 -> [w451]
        tunnel: [w451] -> w424
        tunnel: w423 -> [w450]
        tunnel: [w450] -> w422
        tunnel: w421 -> [w448]
        tunnel: [w447] -> w420
        tunnel: [w446] -> w419
        tunnel: w413 -> [w446]
        tunnel: w424 -> [w459]
        tunnel: w422 -> [w458]
        tunnel: w420 -> [w452]
        tunnel: w419 -> [w453]
        tunnel: [w452] -> w418
        tunnel: [w453] -> w417
        tunnel: [w457] -> w416
        tunnel: [w456] -> w415
        tunnel: w418 -> [w463]
        tunnel: w417 -> [w462]
        tunnel: w416 -> [_]
        tunnel: w415 -> [_]
        frame #0 {
          n77 = call "Shooter_Auto 2.vi"("RunTime"=1.5, "Override?"=FALSE, "Master"=w437) -> ("Master"=w435:T3)  [unwired: 7 in, 1 out]
          n78 = call "Turret Auto.vi"("RunTime"=1.5, "Overide"=FALSE, "Motor1Ref"=w438) -> ("PhoenixMotorControlDevRef"=w436:T3)  [unwired: 8 in]
          n79 = call <vilib>:"WPI_MotorControlSetOutput.vi"("Output"=1.0, "MotorControlDevRef"=w431) -> ("MotorControlDevRef"=w430:T3)  [unwired: 7 in, 2 out]
          n80 = call "Auto_Driving.vi"("MaxTime"=1.5, "Motor2Ref"=w444, "Motor2Distance"=3.0, "Motor1Distance"=3.0, "Motor1Ref"=w445) -> ()  [unwired: 4 in, 3 out]
        }
        frame #1 {
          n81 = call <vilib>:"WPI_MotorControlSetOutput.vi"("Output"=0.85, "MotorControlDevRef"=w448) -> ("MotorControlDevRef"=w447:T3)  [unwired: 7 in, 2 out]
        }
        frame #2 {
          n82 = call "Shooter_Auto 2.vi"("RunTime"=2.75, "Override?"=FALSE, "Master"=w458) -> ("Master"=w456:T3)  [unwired: 7 in, 1 out]
          n83 = call "Turret Auto.vi"("RunTime"=2.75, "Overide"=FALSE, "Motor1Ref"=w459) -> ("PhoenixMotorControlDevRef"=w457:T3)  [unwired: 8 in]
        }
        frame #3 {
          n84 = call <vilib>:"WPI_MotorControlSetOutput.vi"("Output"=0.0, "MotorControlDevRef"=w462) -> ()  [unwired: 7 in, 3 out]
          n85 = call <vilib>:"WPI_MotorControlSetOutput.vi"("Output"=0.0, "MotorControlDevRef"=w463) -> ()  [unwired: 7 in, 3 out]
        }
      }
    }
    frame "3 Ball LL" {
      n86 = flat-sequence {
        tunnel: w474 -> [w498]
        tunnel: w473 -> [w497]
        tunnel: w471 -> [w491]
        tunnel: w472 -> [w490]
        tunnel: [w489] -> w481
        tunnel: [w488] -> w480
        tunnel: w470 -> [w483]
        tunnel: [w482] -> w468
        tunnel: w481 -> [w505]
        tunnel: [w505] -> w479
        tunnel: w480 -> [w504]
        tunnel: [w504] -> w478
        tunnel: [w499] -> w477
        tunnel: [w503] -> w469
        tunnel: w468 -> [w503]
        tunnel: w466 -> [w500]
        tunnel: w479 -> [w514]
        tunnel: w478 -> [w513]
        tunnel: w477 -> [w510]
        tunnel: [w506] -> w476
        tunnel: [w510] -> w475
        tunnel: w469 -> [w509]
        tunnel: w467 -> [w507]
        tunnel: w476 -> [w518]
        tunnel: w475 -> [w517]
        frame #0 {
          n87 = call "Shooter_Auto 2.vi"("RunTime"=2.0, "RPM Override"=15000.0, "Override?"=TRUE, "Followers"=w483, "Master"=w490) -> ("Follower"=w482:T3, "Master"=w488:T3)  [unwired: 5 in]
          n88 = call "Turret Auto.vi"("RunTime"=2.0, "Override_Value"=1240.0, "Overide"=TRUE, "Motor1Ref"=w491) -> ("PhoenixMotorControlDevRef"=w489:T3)  [unwired: 7 in]
          n89 = call "Auto_Driving.vi"("MaxTime"=2.0, "Motor2Ref"=w497, "Motor2Distance"=4.25, "Motor1Distance"=4.25, "Motor1Ref"=w498) -> ()  [unwired: 4 in, 3 out]
        }
        frame #1 {
          n90 = Wait (ms)(milliseconds to wait=u32 1000 ("millisecond timer value")) -> ()  [unwired: 1 out]
          n91 = call <vilib>:"WPI_MotorControlSetOutput.vi"("Output"=1.0, "MotorControlDevRef"=w500) -> ("MotorControlDevRef"=w499:T3)  [unwired: 7 in, 2 out]
        }
        frame #2 {
          n92 = call <vilib>:"WPI_MotorControlSetOutput.vi"("Output"=0.85, "MotorControlDevRef"=w507) -> ("MotorControlDevRef"=w506:T3)  [unwired: 7 in, 2 out]
          n93 = call "Shooter_Auto 2.vi"("RunTime"=2.75, "Override?"=FALSE, "Followers"=w509, "Master"=w513) -> ()  [unwired: 6 in, 2 out]
          n94 = call "Turret Auto.vi"("RunTime"=2.75, "Overide"=FALSE, "Motor1Ref"=w514) -> ()  [unwired: 8 in, 1 out]
        }
        frame #3 {
          n95 = call <vilib>:"WPI_MotorControlSetOutput.vi"("Output"=0.0, "MotorControlDevRef"=w517) -> ()  [unwired: 7 in, 3 out]
          n96 = call <vilib>:"WPI_MotorControlSetOutput.vi"("Output"=0.0, "MotorControlDevRef"=w518) -> ()  [unwired: 7 in, 3 out]
        }
      }
    }
    frame "5 LT" {
      n97 = flat-sequence {
        tunnel: w523 -> [w585]
        tunnel: w575 -> [w583]
        tunnel: w574 -> [w576]
        tunnel: w573 -> [w577]
        tunnel: [w582] -> w572
        tunnel: [w581] -> w571
        tunnel: [w580] -> w570
        tunnel: w569 -> [w580]
        tunnel: w565 -> [w579]
        tunnel: [w579] -> w564
        tunnel: [w578] -> w563
        tunnel: w562 -> [w578]
        tunnel: [w577] -> w522
        tunnel: [w576] -> w521
        tunnel: w572 -> [w590]
        tunnel: w571 -> [w589]
        tunnel: [w595] -> w552
        tunnel: [w594] -> w551
        tunnel: [w593] -> w550
        tunnel: w570 -> [w593]
        tunnel: w564 -> [w592]
        tunnel: [w592] -> w549
        tunnel: [w591] -> w548
        tunnel: w563 -> [w591]
        tunnel: [w590] -> w530
        tunnel: [w589] -> w526
        tunnel: w522 -> [w588]
        tunnel: w521 -> [w587]
        tunnel: w552 -> [w600]
        tunnel: w551 -> [w599]
        tunnel: [w607] -> w547
        tunnel: [w606] -> w546
        tunnel: [w605] -> w545
        tunnel: w550 -> [w605]
        tunnel: w549 -> [w604]
        tunnel: [w604] -> w544
        tunnel: [w603] -> w543
        tunnel: w548 -> [w603]
        tunnel: [w602] -> w531
        tunnel: w530 -> [w602]
        tunnel: [w601] -> w527
        tunnel: w526 -> [w601]
        tunnel: w547 -> [w616]
        tunnel: [w614] -> w542
        tunnel: w546 -> [w615]
        tunnel: [w613] -> w540
        tunnel: w545 -> [w622]
        tunnel: [w622] -> w538
        tunnel: w544 -> [w621]
        tunnel: [w621] -> w536
        tunnel: w543 -> [w620]
        tunnel: [w620] -> w534
        tunnel: [w612] -> w532
        tunnel: w531 -> [w612]
        tunnel: [w611] -> w528
        tunnel: w527 -> [w611]
        tunnel: w542 -> [w624]
        tunnel: [w624] -> w541
        tunnel: w540 -> [w623]
        tunnel: [w623] -> w539
        tunnel: w538 -> [w626]
        tunnel: [w626] -> w537
        tunnel: w536 -> [w629]
        tunnel: [w629] -> w535
        tunnel: w534 -> [w628]
        tunnel: [w628] -> w533
        tunnel: w532 -> [w627]
        tunnel: [w627] -> w529
        tunnel: w528 -> [w625]
        tunnel: [w625] -> w524
        tunnel: w541 -> [w649]
        tunnel: w539 -> [w648]
        tunnel: w537 -> [w645]
        tunnel: [w643] -> w561
        tunnel: [w641] -> w559
        tunnel: [w638] -> w556
        tunnel: w535 -> [w635]
        tunnel: w533 -> [w634]
        tunnel: [w632] -> w554
        tunnel: w529 -> [w631]
        tunnel: [w630] -> w525
        tunnel: w524 -> [w630]
        tunnel: w561 -> [w660]
        tunnel: [w660] -> w560
        tunnel: w559 -> [w659]
        tunnel: [w659] -> w558
        tunnel: [w654] -> w557
        tunnel: w556 -> [w658]
        tunnel: [w658] -> w555
        tunnel: w554 -> [w657]
        tunnel: w553 -> [w655]
        tunnel: w525 -> [w651]
        tunnel: w568 -> [w670]
        tunnel: [w664] -> w567
        tunnel: [w669] -> w566
        tunnel: w560 -> [w665]
        tunnel: w558 -> [w666]
        tunnel: w557 -> [w664]
        tunnel: w555 -> [w661]
        tunnel: w567 -> [w673]
        tunnel: w566 -> [w672]
        frame #0 {
          n98 = call <vilib>:"WPI_MotorControlSetOutput.vi"("Output"=-1.0, "MotorControlDevRef"=w585) -> ("MotorControlDevRef"=w582:T3)  [unwired: 7 in, 2 out]
          n99 = call-poly <vilib>:"WPI_SolenoidSet.vi"("Value"=WPI_SolenoidValue."Reverse", "SolenoidDevRef"=w583) -> ("SolenoidDevRef"=w581:T8)  [unwired: 8 in, 1 out]
        }
        frame #1 {
          n100 = call "Auto_Driving.vi"("MaxTime"=2.35, "Motor2Ref"=w588, "Motor2Distance"=5.7, "Motor1Distance"=5.7, "Motor1Ref"=w587) -> ("Motor Bottom Out"=w594:T3, "Motor Top Out"=w595:T3)  [unwired: 4 in, 1 out]
        }
        frame #2 {
          n101 = call "Auto_Driving.vi"("MaxTime"=1.25, "Motor2Ref"=w599, "Motor2Distance"=-1.22, "Motor1Distance"=1.22, "Motor1Ref"=w600) -> ("Motor Bottom Out"=w606:T3, "Motor Top Out"=w607:T3)  [unwired: 4 in, 1 out]
        }
        frame #3 {
          n102 = call "Auto_Driving.vi"("MaxTime"=2.35, "Motor2Ref"=w615, "Motor2Distance"=4.5, "Motor1Distance"=4.5, "Motor1Ref"=w616) -> ("Motor Bottom Out"=w613:T3, "Motor Top Out"=w614:T3)  [unwired: 4 in, 1 out]
        }
        frame #4 {
        }
        frame #5 {
          n103 = call "Auto_Driving.vi"("MaxTime"=2.5, "Motor2Ref"=w648, "Motor2Distance"=-20.0, "Motor1Distance"=-20.0, "Motor1Ref"=w649) -> ()  [unwired: 4 in, 3 out]
          n104 = call "Turret Auto.vi"("RunTime"=2.35, "Override_Value"=-2100.0, "Overide"=TRUE, "Motor1Ref"=w645) -> ("PhoenixMotorControlDevRef"=w643:T3)  [unwired: 7 in]
          n105 = call <vilib>:"WPI_MotorControlSetOutput.vi"("Output"=-1.0, "MotorControlDevRef"=w631) -> ("MotorControlDevRef"=w632:T3)  [unwired: 7 in, 2 out]
          n106 = call "Shooter_Auto 2.vi"("RunTime"=2.35, "RPM Override"=14000.0, "Override?"=TRUE, "Followers"=w634, "Master"=w635) -> ("Follower"=w638:T3, "Master"=w641:T3)  [unwired: 5 in]
        }
        frame #6 {
          # "Kicker"
          n107 = call <vilib>:"WPI_MotorControlSetOutput.vi"("Output"=1.0, "MotorControlDevRef"=w655) -> ("MotorControlDevRef"=w654:T3)  [unwired: 7 in, 2 out]
          n108 = call <vilib>:"WPI_MotorControlSetOutput.vi"("Output"=0.0, "MotorControlDevRef"=w657) -> ()  [unwired: 7 in, 3 out]
          n109 = call-poly <vilib>:"WPI_SolenoidSet.vi"("Value"=WPI_SolenoidValue."Forward", "SolenoidDevRef"=w651) -> ()  [unwired: 8 in, 2 out]
        }
        frame #7 {
          # "Belting"
          n110 = call "Turret Auto.vi"("RunTime"=3.0, "Overide"=FALSE, "Motor1Ref"=w665) -> ()  [unwired: 8 in, 1 out]
          n111 = call "Shooter_Auto 2.vi"("RunTime"=3.0, "Override?"=FALSE, "Followers"=w661, "Master"=w666) -> ()  [unwired: 6 in, 2 out]
          n112 = call <vilib>:"WPI_MotorControlSetOutput.vi"("Output"=0.85, "MotorControlDevRef"=w670) -> ("MotorControlDevRef"=w669:T3)  [unwired: 7 in, 2 out]
        }
        frame #8 {
          # "Kicker"
          # "Belting"
          n113 = call <vilib>:"WPI_MotorControlSetOutput.vi"("Output"=0.0, "MotorControlDevRef"=w673) -> ()  [unwired: 7 in, 3 out]
          n114 = call <vilib>:"WPI_MotorControlSetOutput.vi"("Output"=0.0, "MotorControlDevRef"=w672) -> ()  [unwired: 7 in, 3 out]
        }
        frame #9 {
        }
        frame #10 {
        }
      }
    }
    frame "7 LT" {
      n115 = flat-sequence {
        tunnel: [w768] -> w751
        tunnel: [w767] -> w750
        tunnel: [w762] -> w749
        tunnel: [w761] -> w748
        tunnel: w720 -> [w760]
        tunnel: w719 -> [w759]
        tunnel: w718 -> [w758]
        tunnel: w717 -> [w757]
        tunnel: [w756] -> w711
        tunnel: w710 -> [w756]
        tunnel: [w755] -> w703
        tunnel: w702 -> [w755]
        tunnel: [w754] -> w697
        tunnel: w696 -> [w754]
        tunnel: [w753] -> w691
        tunnel: w690 -> [w753]
        tunnel: [w752] -> w685
        tunnel: w684 -> [w752]
        tunnel: w751 -> [w779]
        tunnel: w750 -> [w778]
        tunnel: [w781] -> w747
        tunnel: [w780] -> w746
        tunnel: [w779] -> w745
        tunnel: [w778] -> w744
        tunnel: w749 -> [w777]
        tunnel: w748 -> [w776]
        tunnel: [w775] -> w712
        tunnel: w711 -> [w775]
        tunnel: [w774] -> w704
        tunnel: w703 -> [w774]
        tunnel: [w773] -> w698
        tunnel: w697 -> [w773]
        tunnel: [w772] -> w692
        tunnel: w691 -> [w772]
        tunnel: [w771] -> w686
        tunnel: w685 -> [w771]
        tunnel: w747 -> [w795]
        tunnel: w746 -> [w791]
        tunnel: [w801] -> w743
        tunnel: [w800] -> w742
        tunnel: [w799] -> w741
        tunnel: w745 -> [w799]
        tunnel: [w798] -> w740
        tunnel: w744 -> [w798]
        tunnel: [w789] -> w713
        tunnel: w712 -> [w789]
        tunnel: [w788] -> w705
        tunnel: w704 -> [w788]
        tunnel: [w787] -> w699
        tunnel: w698 -> [w787]
        tunnel: [w786] -> w693
        tunnel: w692 -> [w786]
        tunnel: [w785] -> w687
        tunnel: w686 -> [w785]
        tunnel: w743 -> [w815]
        tunnel: [w813] -> w739
        tunnel: w742 -> [w814]
        tunnel: [w812] -> w738
        tunnel: [w811] -> w737
        tunnel: w741 -> [w811]
        tunnel: [w810] -> w736
        tunnel: w740 -> [w810]
        tunnel: [w809] -> w714
        tunnel: w713 -> [w809]
        tunnel: [w808] -> w706
        tunnel: w705 -> [w808]
        tunnel: [w807] -> w700
        tunnel: w699 -> [w807]
        tunnel: [w806] -> w694
        tunnel: w693 -> [w806]
        tunnel: [w805] -> w688
        tunnel: w687 -> [w805]
        tunnel: w739 -> [w825]
        tunnel: [w824] -> w735
        tunnel: w738 -> [w827]
        tunnel: [w826] -> w734
        tunnel: w737 -> [w833]
        tunnel: [w833] -> w733
        tunnel: w736 -> [w832]
        tunnel: [w832] -> w732
        tunnel: [w823] -> w715
        tunnel: w714 -> [w823]
        tunnel: [w822] -> w707
        tunnel: w706 -> [w822]
        tunnel: [w821] -> w701
        tunnel: w700 -> [w821]
        tunnel: [w820] -> w695
        tunnel: w694 -> [w820]
        tunnel: [w819] -> w689
        tunnel: w688 -> [w819]
        tunnel: w735 -> [w857]
        tunnel: w734 -> [w856]
        tunnel: [w852] -> w731
        tunnel: [w850] -> w730
        tunnel: [w847] -> w729
        tunnel: [w843] -> w728
        tunnel: w733 -> [w842]
        tunnel: [w841] -> w727
        tunnel: w732 -> [w841]
        tunnel: [w840] -> w716
        tunnel: w715 -> [w840]
        tunnel: [w839] -> w708
        tunnel: w707 -> [w839]
        tunnel: w701 -> [w838]
        tunnel: w695 -> [w837]
        tunnel: w689 -> [w836]
        tunnel: [w835] -> w681
        tunnel: [w834] -> w678
        tunnel: w731 -> [w871]
        tunnel: [w871] -> w726
        tunnel: w730 -> [w870]
        tunnel: [w870] -> w725
        tunnel: [w866] -> w724
        tunnel: w729 -> [w869]
        tunnel: [w869] -> w723
        tunnel: w728 -> [w868]
        tunnel: w727 -> [w863]
        tunnel: w716 -> [w862]
        tunnel: [w861] -> w709
        tunnel: w708 -> [w861]
        tunnel: [w860] -> w682
        tunnel: w681 -> [w860]
        tunnel: [w859] -> w679
        tunnel: w678 -> [w859]
        tunnel: [w878] -> w722
        tunnel: [w883] -> w721
        tunnel: w726 -> [w879]
        tunnel: w725 -> [w880]
        tunnel: w724 -> [w878]
        tunnel: w723 -> [w875]
        tunnel: w709 -> [w874]
        tunnel: [w873] -> w683
        tunnel: w682 -> [w873]
        tunnel: [w872] -> w680
        tunnel: w679 -> [w872]
        tunnel: w722 -> [w894]
        tunnel: w721 -> [w893]
        tunnel: w683 -> [w888]
        tunnel: w680 -> [w887]
        tunnel: [w886] -> w677
        tunnel: [w885] -> w676
        tunnel: w677 -> [w898]
        tunnel: w676 -> [w897]
        frame #0 {
          n116 = call <vilib>:"WPI_MotorControlSetOutput.vi"("Output"=-1.0, "MotorControlDevRef"=w757) -> ("MotorControlDevRef"=w768:T3)  [unwired: 7 in, 2 out]
          n117 = call <vilib>:"CTRE_Phoenix_MotorControl_ConfigClosedLoopPeakOutput.vi"("slotIdx"=0, "peakOutput"=0.75, "PhoenixMotorControlDevRef"=w760) -> ("PhoenixMotorControlDevRef"=w762:T3)  [unwired: 7 in, 1 out]
          n118 = call <vilib>:"CTRE_Phoenix_MotorControl_ConfigClosedLoopPeakOutput.vi"("slotIdx"=0, "peakOutput"=0.75, "PhoenixMotorControlDevRef"=w759) -> ("PhoenixMotorControlDevRef"=w761:T3)  [unwired: 7 in, 1 out]
          n119 = call-poly <vilib>:"WPI_SolenoidSet.vi"("Value"=WPI_SolenoidValue."Reverse", "SolenoidDevRef"=w758) -> ("SolenoidDevRef"=w767:T8)  [unwired: 8 in, 1 out]
        }
        frame #1 {
          n120 = call "Auto_Driving.vi"("MaxTime"=2.35, "Motor2Ref"=w777, "Motor2Distance"=5.7, "Motor1Distance"=5.7, "Motor1Ref"=w776) -> ("Motor Bottom Out"=w780:T3, "Motor Top Out"=w781:T3)  [unwired: 4 in, 1 out]
        }
        frame #2 {
          n121 = call <vilib>:"CTRE_Phoenix_MotorControl_ConfigClosedLoopPeakOutput.vi"("slotIdx"=0, "peakOutput"=0.5, "PhoenixMotorControlDevRef"=w795) -> ("PhoenixMotorControlDevRef"=w794:T3)  [unwired: 7 in, 1 out]
          n122 = call <vilib>:"CTRE_Phoenix_MotorControl_ConfigClosedLoopPeakOutput.vi"("slotIdx"=0, "peakOutput"=0.5, "PhoenixMotorControlDevRef"=w791) -> ("PhoenixMotorControlDevRef"=w790:T3)  [unwired: 7 in, 1 out]
          n123 = call "Auto_Driving.vi"("MaxTime"=1.25, "Motor2Ref"=w790, "Motor2Distance"=-1.22, "Motor1Distance"=1.22, "Motor1Ref"=w794) -> ("Motor Bottom Out"=w800:T3, "Motor Top Out"=w801:T3)  [unwired: 4 in, 1 out]
        }
        frame #3 {
          n124 = call "Auto_Driving.vi"("MaxTime"=2.35, "Motor2Ref"=w814, "Motor2Distance"=4.5, "Motor1Distance"=4.5, "Motor1Ref"=w815) -> ("Motor Bottom Out"=w812:T3, "Motor Top Out"=w813:T3)  [unwired: 4 in, 1 out]
        }
        frame #4 {
          n125 = call <vilib>:"CTRE_Phoenix_MotorControl_ConfigClosedLoopPeakOutput.vi"("slotIdx"=0, "peakOutput"=0.75, "PhoenixMotorControlDevRef"=w825) -> ("PhoenixMotorControlDevRef"=w824:T3)  [unwired: 7 in, 1 out]
          n126 = call <vilib>:"CTRE_Phoenix_MotorControl_ConfigClosedLoopPeakOutput.vi"("slotIdx"=0, "peakOutput"=0.75, "PhoenixMotorControlDevRef"=w827) -> ("PhoenixMotorControlDevRef"=w826:T3)  [unwired: 7 in, 1 out]
        }
        frame #5 {
          n127 = call "Auto_Driving.vi"("MaxTime"=2.5, "Motor2Ref"=w856, "Motor2Distance"=-20.0, "Motor1Distance"=-20.0, "Motor1Ref"=w857) -> ("Motor Bottom Out"=w835:T3, "Motor Top Out"=w834:T3)  [unwired: 4 in, 1 out]
          n128 = call "Turret Auto.vi"("RunTime"=2.35, "Override_Value"=-2100.0, "Overide"=TRUE, "Motor1Ref"=w836) -> ("PhoenixMotorControlDevRef"=w852:T3)  [unwired: 7 in]
          n129 = call <vilib>:"WPI_MotorControlSetOutput.vi"("Output"=-1.0, "MotorControlDevRef"=w842) -> ("MotorControlDevRef"=w843:T3)  [unwired: 7 in, 2 out]
          n130 = call "Shooter_Auto 2.vi"("RunTime"=2.35, "RPM Override"=14000.0, "Override?"=TRUE, "Followers"=w837, "Master"=w838) -> ("Follower"=w847:T3, "Master"=w850:T3)  [unwired: 5 in]
        }
        frame #6 {
          # "Kicker"
          n131 = call <vilib>:"WPI_MotorControlSetOutput.vi"("Output"=1.0, "MotorControlDevRef"=w862) -> ("MotorControlDevRef"=w866:T3)  [unwired: 7 in, 2 out]
          n132 = call <vilib>:"WPI_MotorControlSetOutput.vi"("Output"=0.0, "MotorControlDevRef"=w868) -> ()  [unwired: 7 in, 3 out]
          n133 = call-poly <vilib>:"WPI_SolenoidSet.vi"("Value"=WPI_SolenoidValue."Forward", "SolenoidDevRef"=w863) -> ()  [unwired: 8 in, 2 out]
        }
        frame #7 {
          # "Belting"
          n134 = call "Turret Auto.vi"("RunTime"=3.0, "Overide"=FALSE, "Motor1Ref"=w879) -> ()  [unwired: 8 in, 1 out]
          n135 = call "Shooter_Auto 2.vi"("RunTime"=3.0, "Override?"=FALSE, "Followers"=w875, "Master"=w880) -> ()  [unwired: 6 in, 2 out]
          n136 = call <vilib>:"WPI_MotorControlSetOutput.vi"("Output"=0.85, "MotorControlDevRef"=w874) -> ("MotorControlDevRef"=w883:T3)  [unwired: 7 in, 2 out]
        }
        frame #8 {
          # "Kicker"
          # "Belting"
          n137 = call <vilib>:"WPI_MotorControlSetOutput.vi"("Output"=0.0, "MotorControlDevRef"=w894) -> ()  [unwired: 7 in, 3 out]
          n138 = call <vilib>:"WPI_MotorControlSetOutput.vi"("Output"=0.0, "MotorControlDevRef"=w893) -> ()  [unwired: 7 in, 3 out]
          n139 = call <vilib>:"CTRE_Phoenix_MotorControl_ConfigClosedLoopPeakOutput.vi"("slotIdx"=0, "peakOutput"=0.5, "PhoenixMotorControlDevRef"=w887) -> ("PhoenixMotorControlDevRef"=w886:T3)  [unwired: 7 in, 1 out]
          n140 = call <vilib>:"CTRE_Phoenix_MotorControl_ConfigClosedLoopPeakOutput.vi"("slotIdx"=0, "peakOutput"=0.5, "PhoenixMotorControlDevRef"=w888) -> ("PhoenixMotorControlDevRef"=w885:T3)  [unwired: 7 in, 1 out]
        }
        frame #9 {
          n141 = call "Auto_Driving.vi"("MaxTime"=2.5, "Motor2Ref"=w897, "Motor2Distance"=1.22, "Motor1Distance"=-1.22, "Motor1Ref"=w898) -> ()  [unwired: 4 in, 3 out]
        }
        frame #10 {
        }
      }
    }
    frame "Six Switch" {
      n142 = flat-sequence {
        tunnel: [w968] -> w950
        tunnel: [w967] -> w949
        tunnel: [w963] -> w948
        tunnel: w943 -> [w962]
        tunnel: w942 -> [w961]
        tunnel: w941 -> [w960]
        tunnel: w940 -> [w959]
        tunnel: w939 -> [w958]
        tunnel: [w957] -> w938
        tunnel: w937 -> [w956]
        tunnel: [w955] -> w934
        tunnel: [w954] -> w932
        tunnel: [w953] -> w930
        tunnel: w929 -> [w953]
        tunnel: [w952] -> w927
        tunnel: w926 -> [w952]
        tunnel: w950 -> [w984]
        tunnel: [w984] -> w921
        tunnel: w949 -> [w983]
        tunnel: [w983] -> w919
        tunnel: [w981] -> w917
        tunnel: [w980] -> w915
        tunnel: w948 -> [w980]
        tunnel: [w979] -> w913
        tunnel: w938 -> [w979]
        tunnel: w936 -> [w978]
        tunnel: [w977] -> w911
        tunnel: w934 -> [w977]
        tunnel: [w976] -> w909
        tunnel: w932 -> [w976]
        tunnel: [w975] -> w907
        tunnel: w930 -> [w975]
        tunnel: [w974] -> w905
        tunnel: w927 -> [w974]
        tunnel: w921 -> [w994]
        tunnel: [w994] -> w920
        tunnel: w919 -> [w993]
        tunnel: [w993] -> w918
        tunnel: w917 -> [w992]
        tunnel: [w992] -> w916
        tunnel: w915 -> [w991]
        tunnel: [w991] -> w914
        tunnel: w913 -> [w990]
        tunnel: [w990] -> w912
        tunnel: w911 -> [w989]
        tunnel: [w989] -> w910
        tunnel: w909 -> [w988]
        tunnel: [w988] -> w908
        tunnel: w907 -> [w987]
        tunnel: [w987] -> w906
        tunnel: w905 -> [w986]
        tunnel: [w986] -> w904
        tunnel: w920 -> [w1008]
        tunnel: w918 -> [w1007]
        tunnel: w916 -> [w1001]
        tunnel: w914 -> [w1002]
        tunnel: [w1001] -> w947
        tunnel: [w1002] -> w946
        tunnel: [w1006] -> w945
        tunnel: [w1005] -> w944
        tunnel: w912 -> [w1000]
        tunnel: [w999] -> w935
        tunnel: w910 -> [w999]
        tunnel: [w998] -> w933
        tunnel: w908 -> [w998]
        tunnel: [w997] -> w931
        tunnel: w906 -> [w997]
        tunnel: [w996] -> w928
        tunnel: w904 -> [w996]
        tunnel: [w995] -> w902
        tunnel: w947 -> [w1026]
        tunnel: w946 -> [w1025]
        tunnel: w945 -> [w1012]
        tunnel: w944 -> [w1013]
        tunnel: w935 -> [w1021]
        tunnel: w933 -> [w1020]
        tunnel: w931 -> [w1018]
        tunnel: w928 -> [w1016]
        tunnel: [w1015] -> w925
        tunnel: [w1014] -> w924
        tunnel: [w1013] -> w923
        tunnel: [w1012] -> w922
        tunnel: [w1011] -> w903
        tunnel: w902 -> [w1011]
        tunnel: w925 -> [w1037]
        tunnel: w924 -> [w1036]
        tunnel: w923 -> [w1031]
        tunnel: w922 -> [w1030]
        tunnel: w903 -> [w1029]
        frame #0 {
          n143 = call "Shooter_Auto 2.vi"("RunTime"=1.5, "RPM Override"=14000.0, "Override?"=TRUE, "Followers"=w962, "Master"=w961) -> ("Follower"=w957:T3, "Master"=w967:T3)  [unwired: 5 in]
          n144 = call "Turret Auto.vi"("RunTime"=1.5, "Overide"=FALSE, "Motor1Ref"=w958) -> ("PhoenixMotorControlDevRef"=w968:T3)  [unwired: 8 in]
          n145 = call <vilib>:"WPI_MotorControlSetOutput.vi"("Output"=1.0, "MotorControlDevRef"=w956) -> ("MotorControlDevRef"=w963:T3)  [unwired: 7 in, 2 out]
          n146 = call "Auto_Driving.vi"("MaxTime"=1.5, "Motor2Ref"=w960, "Motor2Distance"=7.5, "Motor1Distance"=7.5, "Motor1Ref"=w959) -> ("Motor Bottom Out"=w954:T3, "Motor Top Out"=w955:T3)  [unwired: 4 in, 1 out]
        }
        frame #1 {
          n147 = call <vilib>:"WPI_MotorControlSetOutput.vi"("Output"=0.85, "MotorControlDevRef"=w978) -> ("MotorControlDevRef"=w981:T3)  [unwired: 7 in, 2 out]
        }
        frame #2 {
          n148 = Wait (ms)(milliseconds to wait=u32 250) -> ()  [unwired: 1 out]
        }
        frame #3 {
          n149 = call "Shooter_Auto 2.vi"("RunTime"=2.0, "Override?"=FALSE, "Followers"=w1000, "Master"=w1007) -> ("Follower"=w995:T3, "Master"=w1005:T3)  [unwired: 6 in]
          n150 = call "Turret Auto.vi"("RunTime"=2.0, "Overide"=FALSE, "Motor1Ref"=w1008) -> ("PhoenixMotorControlDevRef"=w1006:T3)  [unwired: 8 in]
        }
        frame #4 {
          n151 = call "Auto_Driving.vi"("MaxTime"=0.6, "Motor2Ref"=w1020, "Motor2Distance"=1.25, "Motor1Distance"=1.25, "Motor1Ref"=w1021) -> ()  [unwired: 4 in, 3 out]
          n152 = call <vilib>:"WPI_MotorControlSetOutput.vi"("Output"=-1.0, "MotorControlDevRef"=w1018) -> ("MotorControlDevRef"=w1014:T3)  [unwired: 7 in, 2 out]
          n153 = call <vilib>:"WPI_MotorControlSetOutput.vi"("Output"=0.0, "MotorControlDevRef"=w1025) -> ()  [unwired: 7 in, 3 out]
          n154 = call <vilib>:"WPI_MotorControlSetOutput.vi"("Output"=0.0, "MotorControlDevRef"=w1026) -> ()  [unwired: 7 in, 3 out]
          n155 = call-poly <vilib>:"WPI_SolenoidSet.vi"("Value"=WPI_SolenoidValue."Reverse", "SolenoidDevRef"=w1016) -> ("SolenoidDevRef"=w1015:T8)  [unwired: 8 in, 1 out]
        }
        frame #5 {
          n156 = call <vilib>:"WPI_MotorControlSetOutput.vi"("Output"=0.0, "MotorControlDevRef"=w1036) -> ()  [unwired: 7 in, 3 out]
          n157 = call "Shooter_Auto 2.vi"("RunTime"=1.5, "Override?"=FALSE, "Followers"=w1029, "Master"=w1031) -> ()  [unwired: 6 in, 2 out]
          n158 = call "Turret Auto.vi"("RunTime"=1.5, "Overide"=FALSE, "Motor1Ref"=w1030) -> ()  [unwired: 8 in, 1 out]
          n159 = call-poly <vilib>:"WPI_SolenoidSet.vi"("Value"=WPI_SolenoidValue."Forward", "SolenoidDevRef"=w1037) -> ()  [unwired: 8 in, 2 out]
        }
        frame #6 {
        }
      }
    }
    frame "Six RT" {
      n160 = flat-sequence {
        tunnel: w1081 -> [w1086]
        tunnel: w1078 -> [w1101]
        tunnel: w1082 -> [w1084]
        tunnel: w1079 -> [w1103]
        tunnel: w1080 -> [w1102]
        tunnel: w1077 -> [w1099]
        tunnel: [w1098] -> w1076
        tunnel: [w1097] -> w1075
        tunnel: [w1096] -> w1074
        tunnel: [w1095] -> w1073
        tunnel: [w1094] -> w1068
        tunnel: [w1093] -> w1066
        tunnel: [w1092] -> w1064
        tunnel: w1063 -> [w1092]
        tunnel: [w1091] -> w1062
        tunnel: w1061 -> [w1091]
        tunnel: w1076 -> [w1115]
        tunnel: w1075 -> [w1128]
        tunnel: w1074 -> [w1127]
        tunnel: w1073 -> [w1126]
        tunnel: w1072 -> [w1124]
        tunnel: [w1115] -> w1071
        tunnel: [w1123] -> w1070
        tunnel: [w1122] -> w1069
        tunnel: w1068 -> [w1122]
        tunnel: [w1121] -> w1067
        tunnel: w1066 -> [w1121]
        tunnel: [w1120] -> w1065
        tunnel: w1064 -> [w1120]
        tunnel: w1062 -> [w1119]
        tunnel: [w1118] -> w1058
        tunnel: [w1117] -> w1056
        tunnel: [w1116] -> w1054
        tunnel: [w1113] -> w1040
        tunnel: w1071 -> [w1150]
        tunnel: w1070 -> [w1149]
        tunnel: w1069 -> [w1147]
        tunnel: w1067 -> [w1146]
        tunnel: w1065 -> [w1143]
        tunnel: [w1133] -> w1060
        tunnel: [w1141] -> w1059
        tunnel: w1058 -> [w1141]
        tunnel: [w1140] -> w1057
        tunnel: w1056 -> [w1140]
        tunnel: [w1139] -> w1055
        tunnel: w1054 -> [w1139]
        tunnel: [w1138] -> w1053
        tunnel: [w1137] -> w1052
        tunnel: [w1136] -> w1051
        tunnel: [w1135] -> w1050
        tunnel: [w1134] -> w1048
        tunnel: w1040 -> [w1133]
        tunnel: w1060 -> [w1173]
        tunnel: w1059 -> [w1162]
        tunnel: w1057 -> [w1161]
        tunnel: w1055 -> [w1163]
        tunnel: w1053 -> [w1169]
        tunnel: w1052 -> [w1168]
        tunnel: w1051 -> [w1153]
        tunnel: w1050 -> [w1159]
        tunnel: [w1158] -> w1049
        tunnel: w1048 -> [w1158]
        tunnel: [w1157] -> w1047
        tunnel: [w1156] -> w1046
        tunnel: [w1155] -> w1045
        tunnel: [w1154] -> w1042
        tunnel: [w1153] -> w1041
        tunnel: w1049 -> [w1186]
        tunnel: w1047 -> [w1181]
        tunnel: w1046 -> [w1180]
        tunnel: w1045 -> [w1179]
        tunnel: [w1178] -> w1044
        tunnel: [w1177] -> w1043
        tunnel: w1042 -> [w1177]
        tunnel: w1041 -> [w1175]
        tunnel: w1044 -> [w1189]
        tunnel: w1043 -> [w1188]
        frame #0 {
          n161 = call <vilib>:"CTRE_Phoenix_MotorControl_ConfigClosedLoopPeakOutput.vi"("slotIdx"=0, "peakOutput"=0.65, "PhoenixMotorControlDevRef"=w1084) -> ("PhoenixMotorControlDevRef"=w1083:T3)  [unwired: 7 in, 1 out]
          n162 = call <vilib>:"CTRE_Phoenix_MotorControl_ConfigClosedLoopPeakOutput.vi"("slotIdx"=0, "peakOutput"=0.65, "PhoenixMotorControlDevRef"=w1086) -> ("PhoenixMotorControlDevRef"=w1085:T3)  [unwired: 7 in, 1 out]
          n163 = call "Shooter_Auto 2.vi"("RunTime"=1.75, "RPM Override"=14250.0, "Override?"=TRUE, "Followers"=w1102, "Master"=w1103) -> ("Follower"=w1095:T3, "Master"=w1096:T3)  [unwired: 5 in]
          n164 = call <vilib>:"WPI_MotorControlSetOutput.vi"("Output"=1.0, "MotorControlDevRef"=w1099) -> ("MotorControlDevRef"=w1098:T3)  [unwired: 7 in, 2 out]
          n165 = call "Auto_Driving.vi"("MaxTime"=1.75, "Motor2Ref"=w1085, "Motor2Distance"=4.5, "Motor1Distance"=4.5, "Motor1Ref"=w1083) -> ("Motor Bottom Out"=w1093:T3, "Motor Top Out"=w1094:T3)  [unwired: 4 in, 1 out]
          n166 = call "Turret Auto.vi"("RunTime"=1.75, "Override_Value"=-1980.0, "Overide"=TRUE, "Motor1Ref"=w1101) -> ("PhoenixMotorControlDevRef"=w1097:T3)  [unwired: 7 in]
        }
        frame #1 {
          n167 = call "Shooter_Auto 2.vi"("RunTime"=1.75, "Override?"=FALSE, "Followers"=w1126, "Master"=w1127) -> ("Follower"=w1117:T3, "Master"=w1118:T3)  [unwired: 6 in]
          n168 = call <vilib>:"WPI_MotorControlSetOutput.vi"("Output"=0.85, "MotorControlDevRef"=w1124) -> ("MotorControlDevRef"=w1123:T3)  [unwired: 7 in, 2 out]
          n169 = call-poly <vilib>:"WPI_SolenoidSet.vi"("Value"=WPI_SolenoidValue."Reverse", "SolenoidDevRef"=w1119) -> ("SolenoidDevRef"=w1113:T8)  [unwired: 8 in, 1 out]
          n170 = call "Turret Auto.vi"("RunTime"=1.75, "Overide"=FALSE, "Motor1Ref"=w1128) -> ("PhoenixMotorControlDevRef"=w1116:T3)  [unwired: 8 in]
        }
        frame #2 {
          n171 = call <vilib>:"WPI_MotorControlSetOutput.vi"("Output"=0.0, "MotorControlDevRef"=w1150) -> ("MotorControlDevRef"=w1135:T3)  [unwired: 7 in, 2 out]
          n172 = call <vilib>:"WPI_MotorControlSetOutput.vi"("Output"=0.0, "MotorControlDevRef"=w1149) -> ("MotorControlDevRef"=w1134:T3)  [unwired: 7 in, 2 out]
          n173 = call "Auto_Driving.vi"("MaxTime"=2.25, "Motor2Ref"=w1146, "Motor2Distance"=9.5, "Motor1Distance"=9.5, "Motor1Ref"=w1147) -> ("Motor Bottom Out"=w1137:T3, "Motor Top Out"=w1138:T3)  [unwired: 4 in, 1 out]
          n174 = call <vilib>:"WPI_MotorControlSetOutput.vi"("Output"=-1.0, "MotorControlDevRef"=w1143) -> ("MotorControlDevRef"=w1136:T3)  [unwired: 7 in, 2 out]
        }
        frame #3 {
          n175 = call <vilib>:"WPI_MotorControlSetOutput.vi"("Output"=1.0, "MotorControlDevRef"=w1159) -> ("MotorControlDevRef"=w1154:T3)  [unwired: 7 in, 2 out]
          n176 = call "Shooter_Auto 2.vi"("RunTime"=1.75, "Override?"=FALSE, "Followers"=w1161, "Master"=w1162) -> ("Follower"=w1156:T3, "Master"=w1157:T3)  [unwired: 6 in]
          n177 = call "Auto_Driving.vi"("MaxTime"=2.0, "Motor2Ref"=w1168, "Motor2Distance"=-5.0, "Motor1Distance"=-5.0, "Motor1Ref"=w1169) -> ()  [unwired: 4 in, 3 out]
          n178 = call "Turret Auto.vi"("RunTime"=1.75, "Overide"=FALSE, "Motor1Ref"=w1163) -> ("PhoenixMotorControlDevRef"=w1155:T3)  [unwired: 8 in]
          n179 = call-poly <vilib>:"WPI_SolenoidSet.vi"("Value"=WPI_SolenoidValue."Forward", "SolenoidDevRef"=w1173) -> ()  [unwired: 8 in, 2 out]
        }
        frame #4 {
          n180 = call <vilib>:"WPI_MotorControlSetOutput.vi"("Output"=0.0, "MotorControlDevRef"=w1175) -> ()  [unwired: 7 in, 3 out]
          n181 = call <vilib>:"WPI_MotorControlSetOutput.vi"("Output"=0.85, "MotorControlDevRef"=w1186) -> ("MotorControlDevRef"=w1178:T3)  [unwired: 7 in, 2 out]
          n182 = call "Shooter_Auto 2.vi"("RunTime"=3.25, "Override?"=FALSE, "Followers"=w1180, "Master"=w1181) -> ()  [unwired: 6 in, 2 out]
          n183 = call "Turret Auto.vi"("RunTime"=3.25, "Overide"=FALSE, "Motor1Ref"=w1179) -> ()  [unwired: 8 in, 1 out]
        }
        frame #5 {
          n184 = call <vilib>:"WPI_MotorControlSetOutput.vi"("Output"=0.0, "MotorControlDevRef"=w1189) -> ()  [unwired: 7 in, 3 out]
          n185 = call <vilib>:"WPI_MotorControlSetOutput.vi"("Output"=0.0, "MotorControlDevRef"=w1188) -> ()  [unwired: 7 in, 3 out]
        }
        frame #6 {
        }
        frame #7 {
        }
      }
    }
    frame "Eight Ball Extravaganza" {
      n186 = flat-sequence {
        tunnel: w1228 -> [w1278]
        tunnel: w1229 -> [w1276]
        tunnel: [w1275] -> w1268
        tunnel: w1227 -> [w1275]
        tunnel: [w1274] -> w1267
        tunnel: w1226 -> [w1274]
        tunnel: [w1273] -> w1266
        tunnel: [w1272] -> w1265
        tunnel: [w1271] -> w1264
        tunnel: w1230 -> [w1271]
        tunnel: w1232 -> [w1270]
        tunnel: [w1270] -> w1263
        tunnel: [w1269] -> w1262
        tunnel: w1231 -> [w1269]
        tunnel: w1268 -> [w1291]
        tunnel: w1267 -> [w1290]
        tunnel: [w1286] -> w1261
        tunnel: w1266 -> [w1286]
        tunnel: [w1285] -> w1260
        tunnel: w1265 -> [w1285]
        tunnel: [w1284] -> w1259
        tunnel: [w1283] -> w1258
        tunnel: [w1282] -> w1257
        tunnel: w1264 -> [w1282]
        tunnel: w1263 -> [w1281]
        tunnel: [w1281] -> w1256
        tunnel: [w1280] -> w1255
        tunnel: w1262 -> [w1280]
        tunnel: w1261 -> [w1302]
        tunnel: w1260 -> [w1300]
        tunnel: [w1298] -> w1254
        tunnel: w1259 -> [w1298]
        tunnel: [w1297] -> w1253
        tunnel: w1258 -> [w1297]
        tunnel: [w1296] -> w1252
        tunnel: w1257 -> [w1296]
        tunnel: w1256 -> [w1295]
        tunnel: [w1295] -> w1251
        tunnel: [w1294] -> w1250
        tunnel: w1255 -> [w1294]
        tunnel: [w1293] -> w1249
        tunnel: [w1292] -> w1211
        tunnel: w1254 -> [w1311]
        tunnel: w1253 -> [w1310]
        tunnel: [w1309] -> w1248
        tunnel: [w1308] -> w1247
        tunnel: [w1307] -> w1246
        tunnel: w1252 -> [w1307]
        tunnel: w1251 -> [w1306]
        tunnel: [w1306] -> w1245
        tunnel: [w1305] -> w1244
        tunnel: w1250 -> [w1305]
        tunnel: [w1304] -> w1243
        tunnel: w1249 -> [w1304]
        tunnel: [w1303] -> w1212
        tunnel: w1211 -> [w1303]
        tunnel: w1248 -> [w1323]
        tunnel: w1247 -> [w1319]
        tunnel: w1246 -> [w1340]
        tunnel: [w1338] -> w1242
        tunnel: [w1336] -> w1241
        tunnel: [w1333] -> w1240
        tunnel: w1245 -> [w1330]
        tunnel: w1244 -> [w1329]
        tunnel: w1243 -> [w1328]
        tunnel: [w1326] -> w1239
        tunnel: [w1317] -> w1221
        tunnel: [w1316] -> w1218
        tunnel: [w1315] -> w1213
        tunnel: w1212 -> [w1315]
        tunnel: w1242 -> [w1355]
        tunnel: [w1355] -> w1238
        tunnel: w1241 -> [w1354]
        tunnel: [w1354] -> w1237
        tunnel: [w1349] -> w1236
        tunnel: w1240 -> [w1353]
        tunnel: [w1353] -> w1235
        tunnel: w1239 -> [w1352]
        tunnel: w1225 -> [w1350]
        tunnel: [w1347] -> w1222
        tunnel: w1221 -> [w1347]
        tunnel: [w1346] -> w1219
        tunnel: w1218 -> [w1346]
        tunnel: [w1345] -> w1216
        tunnel: [w1344] -> w1214
        tunnel: w1213 -> [w1344]
        tunnel: w1224 -> [w1371]
        tunnel: [w1365] -> w1234
        tunnel: [w1370] -> w1233
        tunnel: w1238 -> [w1366]
        tunnel: w1237 -> [w1367]
        tunnel: w1236 -> [w1365]
        tunnel: w1235 -> [w1362]
        tunnel: [w1361] -> w1223
        tunnel: w1222 -> [w1361]
        tunnel: [w1360] -> w1220
        tunnel: w1219 -> [w1360]
        tunnel: [w1359] -> w1217
        tunnel: w1216 -> [w1359]
        tunnel: [w1358] -> w1215
        tunnel: w1214 -> [w1358]
        tunnel: [w1357] -> w1205
        tunnel: [w1356] -> w1197
        tunnel: w1234 -> [w1393]
        tunnel: w1233 -> [w1392]
        tunnel: w1223 -> [w1385]
        tunnel: w1220 -> [w1384]
        tunnel: w1217 -> [w1380]
        tunnel: w1215 -> [w1379]
        tunnel: [w1380] -> w1210
        tunnel: [w1379] -> w1209
        tunnel: [w1378] -> w1208
        tunnel: [w1377] -> w1207
        tunnel: [w1376] -> w1206
        tunnel: w1205 -> [w1376]
        tunnel: [w1375] -> w1204
        tunnel: [w1374] -> w1199
        tunnel: [w1373] -> w1198
        tunnel: w1197 -> [w1373]
        tunnel: w1210 -> [w1419]
        tunnel: w1209 -> [w1418]
        tunnel: w1208 -> [w1417]
        tunnel: w1207 -> [w1416]
        tunnel: w1206 -> [w1409]
        tunnel: w1204 -> [w1406]
        tunnel: [w1405] -> w1203
        tunnel: [w1404] -> w1202
        tunnel: [w1403] -> w1201
        tunnel: [w1400] -> w1200
        tunnel: w1199 -> [w1400]
        tunnel: w1198 -> [w1399]
        tunnel: [w1398] -> w1196
        tunnel: [w1397] -> w1195
        tunnel: [w1396] -> w1192
        tunnel: w1203 -> [w1432]
        tunnel: w1202 -> [w1431]
        tunnel: w1201 -> [w1430]
        tunnel: w1200 -> [w1428]
        tunnel: w1196 -> [w1425]
        tunnel: w1195 -> [w1424]
        tunnel: [w1423] -> w1194
        tunnel: [w1422] -> w1193
        tunnel: w1192 -> [w1422]
        tunnel: w1194 -> [w1438]
        tunnel: w1193 -> [w1437]
        frame #0 {
          n187 = call <vilib>:"WPI_MotorControlSetOutput.vi"("Output"=-1.0, "MotorControlDevRef"=w1278) -> ("MotorControlDevRef"=w1273:T3)  [unwired: 7 in, 2 out]
          n188 = call-poly <vilib>:"WPI_SolenoidSet.vi"("Value"=WPI_SolenoidValue."Reverse", "SolenoidDevRef"=w1276) -> ("SolenoidDevRef"=w1272:T8)  [unwired: 8 in, 1 out]
        }
        frame #1 {
          n189 = call "Auto_Driving.vi"("MaxTime"=2.35, "Motor2Ref"=w1290, "Motor2Distance"=7.25, "Motor1Distance"=7.25, "Motor1Ref"=w1291) -> ("Motor Bottom Out"=w1283:T3, "Motor Top Out"=w1284:T3)  [unwired: 4 in, 1 out]
        }
        frame #2 {
          n190 = call <vilib>:"WPI_MotorControlSetOutput.vi"("Output"=0.0, "MotorControlDevRef"=w1302) -> ("MotorControlDevRef"=w1293:T3)  [unwired: 7 in, 2 out]
          n191 = call-poly <vilib>:"WPI_SolenoidSet.vi"("Value"=WPI_SolenoidValue."Forward", "SolenoidDevRef"=w1300) -> ("SolenoidDevRef"=w1292:T8)  [unwired: 8 in, 1 out]
        }
        frame #3 {
          n192 = call "Auto_Driving.vi"("MaxTime"=1.25, "Motor2Ref"=w1310, "Motor2Distance"=-1.5, "Motor1Distance"=1.5, "Motor1Ref"=w1311) -> ("Motor Bottom Out"=w1308:T3, "Motor Top Out"=w1309:T3)  [unwired: 4 in, 1 out]
        }
        frame #4 {
          n193 = call <vilib>:"CTRE_Phoenix_MotorControl_ConfigClosedLoopPeakOutput.vi"("slotIdx"=0, "peakOutput"=0.75, "PhoenixMotorControlDevRef"=w1323) -> ("PhoenixMotorControlDevRef"=w1322:T3)  [unwired: 7 in, 1 out]
          n194 = call <vilib>:"CTRE_Phoenix_MotorControl_ConfigClosedLoopPeakOutput.vi"("slotIdx"=0, "peakOutput"=0.75, "PhoenixMotorControlDevRef"=w1319) -> ("PhoenixMotorControlDevRef"=w1318:T3)  [unwired: 7 in, 1 out]
          n195 = call "Turret Auto.vi"("RunTime"=2.35, "Override_Value"=-4225.0, "Overide"=TRUE, "Motor1Ref"=w1340) -> ("PhoenixMotorControlDevRef"=w1338:T3)  [unwired: 7 in]
          n196 = call <vilib>:"WPI_MotorControlSetOutput.vi"("Output"=-1.0, "MotorControlDevRef"=w1328) -> ("MotorControlDevRef"=w1326:T3)  [unwired: 7 in, 2 out]
          n197 = call "Shooter_Auto 2.vi"("RunTime"=2.35, "RPM Override"=14000.0, "Override?"=TRUE, "Followers"=w1329, "Master"=w1330) -> ("Follower"=w1333:T3, "Master"=w1336:T3)  [unwired: 5 in]
          n198 = call "Auto_Driving.vi"("MaxTime"=2.5, "Motor2Ref"=w1318, "Motor2Distance"=-12.0, "Motor1Distance"=-12.0, "Motor1Ref"=w1322) -> ("Motor Bottom Out"=w1317:T3, "Motor Top Out"=w1316:T3)  [unwired: 4 in, 1 out]
        }
        frame #5 {
          # "Kicker"
          n199 = call <vilib>:"WPI_MotorControlSetOutput.vi"("Output"=1.0, "MotorControlDevRef"=w1350) -> ("MotorControlDevRef"=w1349:T3)  [unwired: 7 in, 2 out]
          n200 = call <vilib>:"WPI_MotorControlSetOutput.vi"("Output"=0.0, "MotorControlDevRef"=w1352) -> ("MotorControlDevRef"=w1345:T3)  [unwired: 7 in, 2 out]
        }
        frame #6 {
          # "Belting"
          n201 = call "Turret Auto.vi"("RunTime"=3.0, "Overide"=FALSE, "Motor1Ref"=w1366) -> ("PhoenixMotorControlDevRef"=w1356:T3)  [unwired: 8 in]
          n202 = call "Shooter_Auto 2.vi"("RunTime"=3.0, "Override?"=FALSE, "Followers"=w1362, "Master"=w1367) -> ("Master"=w1357:T3)  [unwired: 6 in, 1 out]
          n203 = call <vilib>:"WPI_MotorControlSetOutput.vi"("Output"=0.85, "MotorControlDevRef"=w1371) -> ("MotorControlDevRef"=w1370:T3)  [unwired: 7 in, 2 out]
        }
        frame #7 {
          # "Kicker"
          # "Belting"
          n204 = call <vilib>:"WPI_MotorControlSetOutput.vi"("Output"=0.0, "MotorControlDevRef"=w1393) -> ("MotorControlDevRef"=w1375:T3)  [unwired: 7 in, 2 out]
          n205 = call <vilib>:"WPI_MotorControlSetOutput.vi"("Output"=0.0, "MotorControlDevRef"=w1392) -> ("MotorControlDevRef"=w1374:T3)  [unwired: 7 in, 2 out]
          n206 = call <vilib>:"CTRE_Phoenix_MotorControl_ConfigClosedLoopPeakOutput.vi"("slotIdx"=0, "peakOutput"=0.5, "PhoenixMotorControlDevRef"=w1384) -> ("PhoenixMotorControlDevRef"=w1386:T3)  [unwired: 7 in, 1 out]
          n207 = call <vilib>:"CTRE_Phoenix_MotorControl_ConfigClosedLoopPeakOutput.vi"("slotIdx"=0, "peakOutput"=0.5, "PhoenixMotorControlDevRef"=w1385) -> ("PhoenixMotorControlDevRef"=w1387:T3)  [unwired: 7 in, 1 out]
          n208 = call "Auto_Driving.vi"("MaxTime"=1.5, "Motor2Ref"=w1387, "Motor2Distance"=-2.5, "Motor1Distance"=2.5, "Motor1Ref"=w1386) -> ("Motor Bottom Out"=w1377:T3, "Motor Top Out"=w1378:T3)  [unwired: 4 in, 1 out]
        }
        frame #8 {
          n209 = call <vilib>:"WPI_MotorControlSetOutput.vi"("Output"=1.0, "MotorControlDevRef"=w1406) -> ("MotorControlDevRef"=w1396:T3)  [unwired: 7 in, 2 out]
          n210 = call <vilib>:"WPI_MotorControlSetOutput.vi"("Output"=-1.0, "MotorControlDevRef"=w1419) -> ("MotorControlDevRef"=w1397:T3)  [unwired: 7 in, 2 out]
          n211 = call "Shooter_Auto 2.vi"("RunTime"=1.5, "RPM Override"=14000.0, "Override?"=TRUE, "Master"=w1409) -> ("Follower"=w1403:T3, "Master"=w1404:T3)  [unwired: 6 in]
          n212 = call "Turret Auto.vi"("RunTime"=1.5, "Override_Value"=0.0, "Overide"=TRUE, "Motor1Ref"=w1399) -> ("PhoenixMotorControlDevRef"=w1405:T3)  [unwired: 7 in]
          n213 = call "Auto_Driving.vi"("MaxTime"=1.5, "Motor2Ref"=w1416, "Motor2Distance"=1.5, "Motor1Distance"=-1.5, "Motor1Ref"=w1417) -> ()  [unwired: 4 in, 3 out]
          n214 = call-poly <vilib>:"WPI_SolenoidSet.vi"("Value"=WPI_SolenoidValue."Reverse", "SolenoidDevRef"=w1418) -> ("SolenoidDevRef"=w1398:T8)  [unwired: 8 in, 1 out]
        }
        frame #9 {
          n215 = call "Shooter_Auto 2.vi"("RunTime"=1.5, "Override?"=FALSE, "Followers"=w1430, "Master"=w1431) -> ()  [unwired: 6 in, 2 out]
          n216 = call <vilib>:"WPI_MotorControlSetOutput.vi"("Output"=0.85, "MotorControlDevRef"=w1428) -> ("MotorControlDevRef"=w1423:T3)  [unwired: 7 in, 2 out]
          n217 = call "Turret Auto.vi"("RunTime"=1.5, "Overide"=FALSE, "Motor1Ref"=w1432) -> ()  [unwired: 8 in, 1 out]
          n218 = call <vilib>:"WPI_MotorControlSetOutput.vi"("Output"=0.0, "MotorControlDevRef"=w1424) -> ()  [unwired: 7 in, 3 out]
          n219 = call-poly <vilib>:"WPI_SolenoidSet.vi"("Value"=WPI_SolenoidValue."Forward", "SolenoidDevRef"=w1425) -> ()  [unwired: 8 in, 2 out]
        }
        frame #10 {
          n220 = call <vilib>:"WPI_MotorControlSetOutput.vi"("Output"=0.0, "MotorControlDevRef"=w1438) -> ()  [unwired: 7 in, 3 out]
          n221 = call <vilib>:"WPI_MotorControlSetOutput.vi"("Output"=0.0, "MotorControlDevRef"=w1437) -> ()  [unwired: 7 in, 3 out]
        }
      }
    }
    frame "PID" {
      n222 = call-poly <vilib>:"CTRE_Phoenix_MotorControl_SetIntegratedSensorPosition_TalonFX_Polymorphic.vi"("New Position"=0.0, "PhoenixMotorControlDevRef"=w1444) -> ("PhoenixMotorControlDevRef"=w1441:T3)  [unwired: 8 in, 1 out]
      n223 = call-poly <vilib>:"CTRE_Phoenix_MotorControl_SetIntegratedSensorPosition_TalonFX_Polymorphic.vi"("New Position"=0.0, "PhoenixMotorControlDevRef"=w1443) -> ("PhoenixMotorControlDevRef"=w1442:T3)  [unwired: 8 in, 1 out]
      n224 = flat-sequence {
        tunnel: w1441 -> [w1450]
        tunnel: w1442 -> [w1451]
        tunnel: [w1451] -> w1448
        tunnel: [w1450] -> w1447
        tunnel: w1448 -> [w1465]
        tunnel: w1447 -> [w1464]
        frame #0 {
          n225 = Wait (ms)(milliseconds to wait=u32 200) -> ()  [unwired: 1 out]
        }
        frame #1 {
          w1453 = T11 0 items=["PercentOutput"=0, "Position"=1, "Velocity"=2, "Current"=3, "Follower"=5, "MotionProfile"=6, "MotionMagic"=7, "MotionProfileArc"=10, "Disabled"=15] ("Control Mode")
          w1456 = T11 0 items=["PercentOutput"=0, "Position"=1, "Velocity"=2, "Current"=3, "Follower"=5, "MotionProfile"=6, "MotionMagic"=7, "MotionProfileArc"=10, "Disabled"=15] ("Control Mode")
          w1468 = T11 1 items=["PercentOutput"=0, "Position"=1, "Velocity"=2, "Current"=3, "Follower"=5, "MotionProfile"=6, "MotionMagic"=7, "MotionProfileArc"=10, "Disabled"=15] ("Control Mode")
          w1470 = T11 1 items=["PercentOutput"=0, "Position"=1, "Velocity"=2, "Current"=3, "Follower"=5, "MotionProfile"=6, "MotionMagic"=7, "MotionProfileArc"=10, "Disabled"=15] ("Control Mode")
          w1467 = 19290.0 ("y")
          # "Ticks per foot\nor\nticks per inch"
          n226 = Multiply(x=5.0 ("Motor1Distance"), y=w1467) -> (x*y=w1469:dbl)
          n227 = call <vilib>:"CTRE_Phoenix_MotorControl_Set.vi"("Output"=w1469, "Control Mode"=w1470, "PhoenixMotorControlDevRef"=w1464) -> ("error out"=w1462:errorcluster, "PhoenixMotorControlDevRef"=w1463:T3)  [unwired: 7 in]
          n228 = Multiply(x=w1467, y=5.0) -> (x*y=w1466:dbl)
          n229 = call <vilib>:"CTRE_Phoenix_MotorControl_Set.vi"("Output"=w1466, "Control Mode"=w1468, "PhoenixMotorControlDevRef"=w1465) -> ("error out"=w1460:errorcluster, "PhoenixMotorControlDevRef"=w1461:T3)  [unwired: 7 in]
          n230 = Tick Count (ms)() -> (millisecond timer value=w1471:u32)
          n231 = while {
            tunnel: w1471 -> [w1482]
            tunnel: w1466 -> [_]
            tunnel: w1469 -> [w1477]
            tunnel: w1461 -> [w1475]
            tunnel: w1460 -> [_]
            tunnel: w1463 -> [w1474]
            tunnel: w1462 -> [_]
            tunnel: [w1475] -> w1454
            tunnel: [w1474] -> w1457
            stop <- w1472 stop-if-true
            # "If within 100 ticks, Stop"
            # "If within 100 ticks, Stop"
            n232 = call-poly <vilib>:"NT Write Value.vi"("Numeric"=w1477, "Name"="DSetPoint") -> ()  [unwired: 9 in, 1 out]
            n233 = Wait (ms)(milliseconds to wait=u32 20) -> ()  [unwired: 1 out]
            n234 = Tick Count (ms)() -> (millisecond timer value=w1483:u32)
            n235 = Subtract(x=w1483, y=w1482) -> (x-y=w1480:u32)
            n236 = Divide(x=w1480, y=1000.0) -> (x/y=w1479:dbl)
            n237 = Greater?(x=w1479, y=5.0) -> (0:w1472:bool)
          }
          n238 = call <vilib>:"CTRE_Phoenix_MotorControl_Set.vi"("Output"=0.0, "Control Mode"=w1453, "PhoenixMotorControlDevRef"=w1454) -> ()  [unwired: 7 in, 2 out]
          n239 = call <vilib>:"CTRE_Phoenix_MotorControl_Set.vi"("Output"=0.0, "Control Mode"=w1456, "PhoenixMotorControlDevRef"=w1457) -> ()  [unwired: 7 in, 2 out]
        }
      }
    }
  }
